vi "main 0.9.2.vi"() -> ()   [LabVIEW 2017]
uses:
  coherent/CH_LM/CH_LM Communication Mode.ctl
  ISEGNHQxxu/iseg NHQ VISA Control.ctl
  <vilib>/Analysis/1siggen.llb/Ramp Pattern by Samples.vi
  <vilib>/Utility/file.llb/Read From Spreadsheet File (DBL).vi
  <vilib>/Instr/_visa.llb/VISA Configure Serial Port (Instr).vi
  Keysight B2980 Series/Public/Data/Read Measurement (Single Point).vi
  Keysight B2980 Series/Public/Configure/Measurement/Configure Current Measurement (Aperture).vi
  <vilib>/Utility/file.llb/Write To Spreadsheet File (DBL).vi
  <vilib>/Utility/file.llb/Write To Spreadsheet File (string).vi
  <vilib>/Platform/browser.llb/Open URL in Default Browser (path).vi
  <vilib>/Analysis/NI_AALBase.lvlib
  coherent/CH_LM.lvlib
  Newport ESP301/Newport ESP301.lvlib
  Keysight B2980 Series/Keysight B2980 Series.lvlib
panel:
  in  "zero":bool
  in  "clear":bool
  in  "Enable Input (F: Disable)":bool
  in  "Enable Output (F: Disable)":bool
  in  "Output Level (0 V)":dbl
  in  "Source Range (20 V)":dbl=20.0
  in  "Aperture Type (1: Medium)":i32(ring)=1 items=["Short", "Medium", "Long"]
  in  "Aperture Integration Time (0.002 s)":dbl=0.002
  in  "Current Range (2E-6 A)":dbl=2e-06
  in  "Auto Current Range (T: Enable)":bool=TRUE
  in  "Auto Current Aperture (T: Enable)":bool=TRUE
  in  "open base path":bool
  in  "Path":path=path "Y:/Ediff/data/2017/01/170106"
  in  "stop":bool
  out "Slide":dbl(slide)=0.99 scale=0.0..1.0
  in  "Tab Control":T1(tab)
  in  "offset":dbl
  out "keysight_graph":cluster{dbl, "mean":dbl}(graph)
  out "esp_pos_fs":dbl caption="[fs]" format="%.6g"
  in  "snap":bool
  in  "dark":bool
  in  "savebin":bool
  in  "savepng":bool
  in  "count?":bool
  in  "dark?":bool=TRUE
  in  "threshold":i32=110
  in  "t_exp":dbl=0.1 caption="exp time [s]"
  in  "dark_load":bool
  in  "frames":i32=100
  in  "avg[t] acc[f]":bool=TRUE
  out "Actual Voltage":dbl[unit]=-0.6 format="%.2f"
  in  "volt_set":bool
  in  "Nominal Voltage":sgl=50.0 max=4000 format="%.2f"
  out "laser power":sgl=6.5658232e-06 format="%^.3e"
  out "Waveform Chart":dbl(graph)=159723533.31
  out "noise-o-meter":dbl=nan format="%.1g"
  in  "array size":i32
  out "[mm]":dbl format="%.6g"
  in  "esp_rel+":bool
  in  "esp_rel-":bool
  in  "esp_abs_go":bool
  in  "esp_rel_delta":dbl=0.1 caption="delta [mm]" min=0.0
  in  "esp_abs_time":dbl caption="[fs]"
  in  "esp_set_t0":bool
  out "t0 @":dbl format="%.6g"
  in  "esp_abs_dest":dbl caption="[mm]"
  in  "Value in":dbl=4.0 caption="binning"
  in  "stats":dbl
  out "x*y":dbl
  in  "x":sgl
  out "Measurement":dbl format="%^#_6g"
  out "e / pulse":dbl
  in  "array size 2":i32
  out "mean":dbl format="%^.2e"
  out "std":dbl format="%^.2e"
  in  "delayscan_go":bool
  in  "waypoints":string[][](table)=[["-100000", "5000"], ["50000", ""], ["", ""]]
  in  "delayscan_header":string="DelayScan01" caption="header"
  in  "iterations":i32
  out "XY Graph":cluster{"Array":dbl[], dbl[]}(graph)
  in  "delayscan_stop":bool
  out "XY Graph 2":cluster{"X":dbl[], "Best Gaussian Fit":dbl[]}[](graph)
  in  "meas_start_power2":bool
  out "meas_voltage":i32=1
  in  "header":string="PowerVoltScan1"
  in  "meas_start_power":bool
  out "meas_power":sgl=6.5658234e-09 format="%.3f"
  in  "powerscan_n":i32
  out "prog":i32
  in  "pause":bool
  in  "Axis":string(combo)
  out "center":dbl
  in  "range+-[nm]":dbl
  in  "n":i32
  in  "rand[t] seq [f]":bool
  in  "zscan?":bool
  out "Slide 2":dbl(slide)=0.999 scale=0.0..1.0
  in  "meas_stop_volt":bool
  in  "meas_start_volt":bool
  in  "head":string="PowerVoltScan1"
  in  "volt_start":dbl format="%0.2f"
  in  "volt_end":dbl=1.0 format="%0.2f"
  in  "volt_samples":i32=128
  in  "move2com":bool
  in  "window2":dbl=10000.0 caption="+/- window" format="%#_6e"
  in  "steps2":u32=21 caption="steps"
  out "XY":dbl[][](graph)
  in  "meas_start_XY":bool
  in  "Axis2":string(combo)="4D Z"
  in  "Axis1":string(combo)="4D Z"
  in  "window1":dbl=10000.0 caption="+/- window" format="%#_6e"
  in  "steps1":u32=21 caption="steps"
  in  "meas_stop_XY":bool
  in  "showcom":bool
  in  "VISA ISEG":refnum<visa-resource-name>="COM6"
  in  "Channel (A)":enum16{"A", "B"}(ring)=enum."B"
  in  "IP address":string="172.24.192.135"
  out "error out":errorcluster
  out "coherent":errorcluster={"status"=TRUE, "code"=-1307, "source"="CH_LM.lvlib:CH_LM FGV Meter Info.vi<ERR>\nMeter index not found.\n\n\n<b>Complete call chain:</b>\r\n     CH_LM.lvlib:CH_LM FGV Meter Info.vi\r\n     CH_LM.lvlib:CH_LM Close.vi\r\n     main 0.9.vi"}
  in  "volt_timeout":u32=6000
  in  "volt_threshold":sgl=2.0 max=4000 format="%.2f"
  in  "esp_axis":i32=2 caption="ESP Axis" min=1 max=3
  in  "esp_visa":refnum<visa-resource-name>="COM1" caption="ESP VISA"
  out "esp301":errorcluster={"status"=TRUE, "code"=-1073807346, "source"="VISA Open in Newport ESP301.lvlib:Initialize.vi->main 0.9.vi"}
  out "response":string
  in  "arduino COM":refnum<visa-resource-name>="COM13"
  in  "arduino_steps":i32
  in  "arduino_go":bool
  out "keysight 2":errorcluster={"status"=TRUE, "code"=-1073807346, "source"="VISA Open in Newport ESP301.lvlib:Initialize.vi->main 0.9.vi"}
  in  "keysight":refnum<visa-resource-name>="USB0::0x0957::0x9418::MY54320162::INSTR"
  in  "Channel (1: Channel 1)":i32(ring)=1 items=["Channel 1"=1, "Channel 2"=2]
  out "captured":dbl[][](graph)
  out "live":dbl[][](graph)
  in  "close":bool
  # "%"
  # "camera"
  # "voltage supply"
  # "delay stage"
  # "absolute"
  # "power meter"
  # "Axis2"
  # "Axis1"
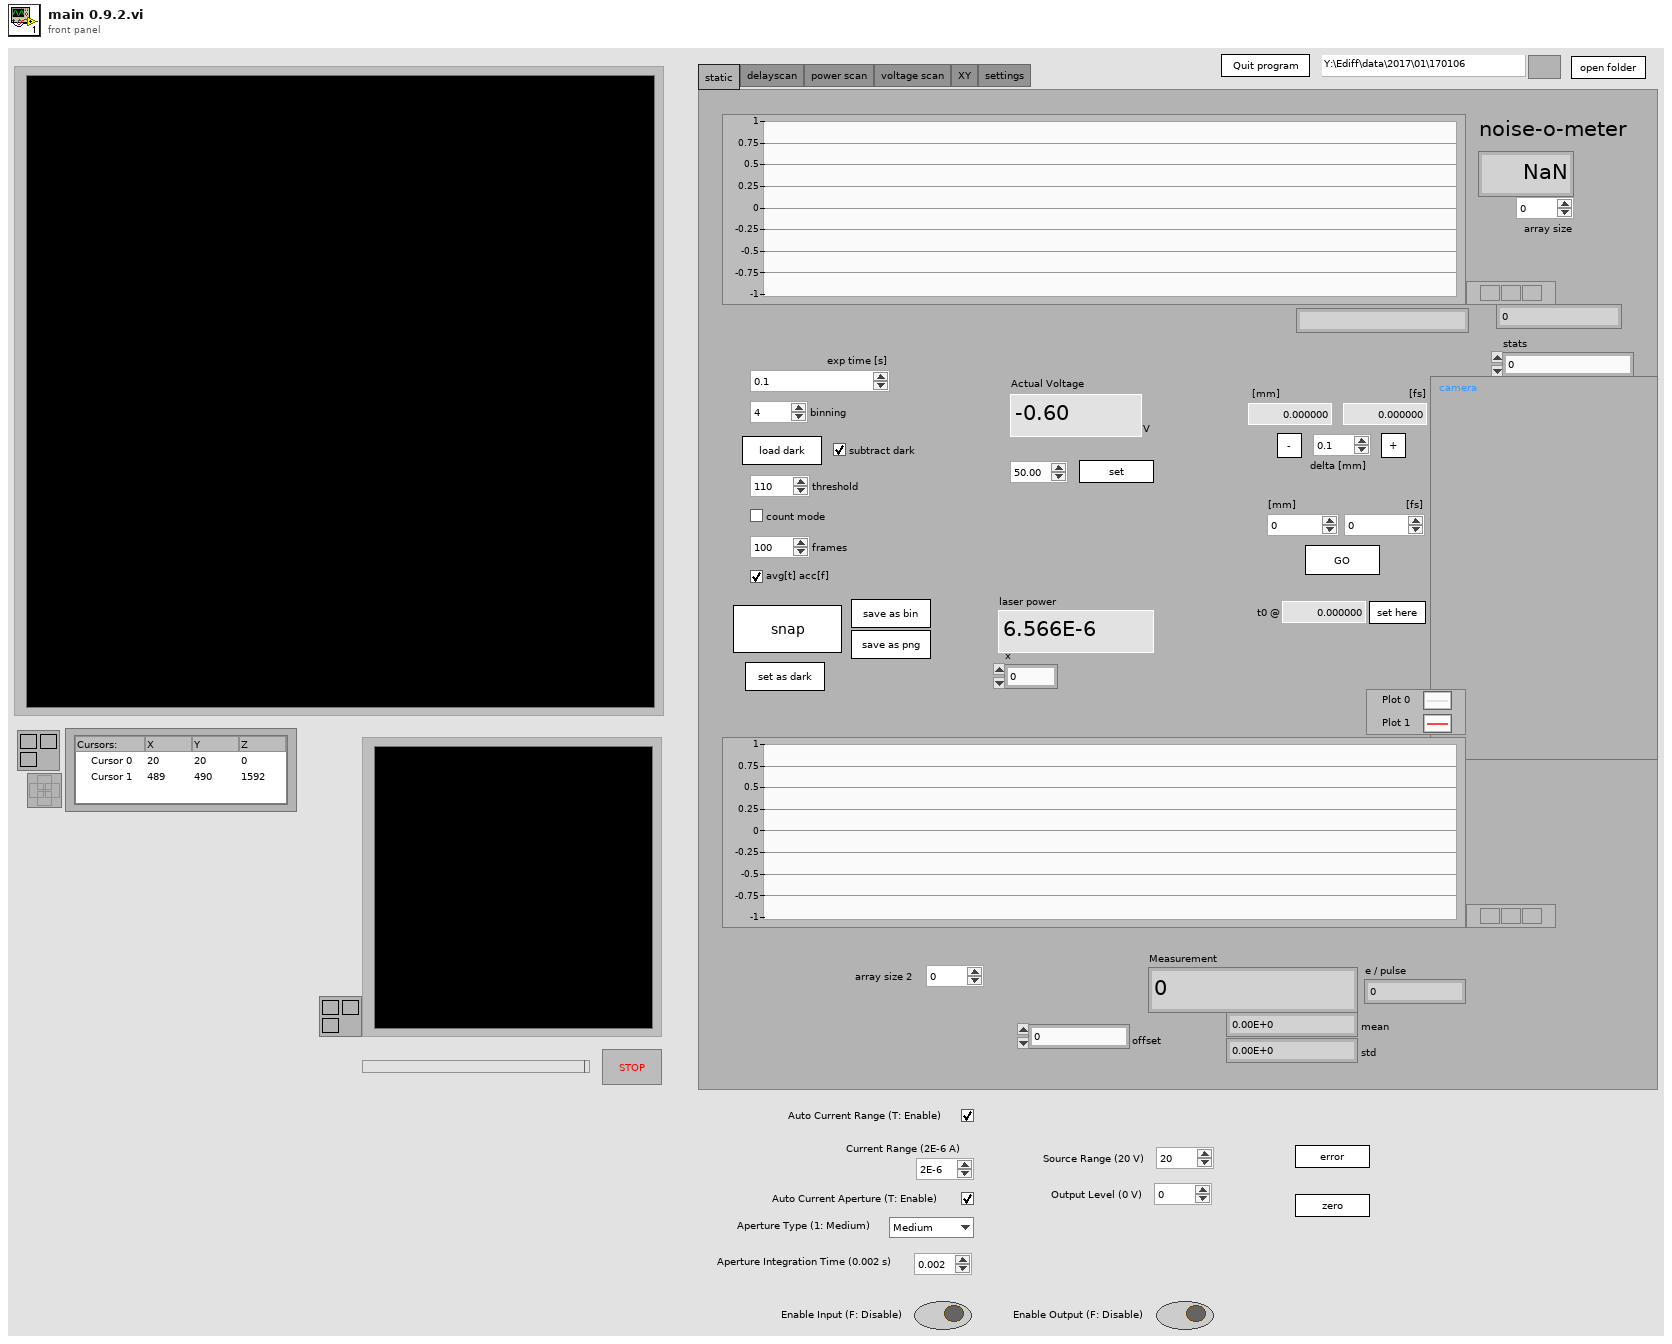
[diagram p1: front panel]
types:
  T1 = enum32{"static", "delayscan", "power scan", "voltage scan", "XY", "settings"}
  T2 = typedef "CH_LM.lvlib/CH_LM Communication Mode.ctl" = enum16{"None", "USB", "GPIB", "RS232"}
  T3 = typedef "Image Type" = u32
  T4 = typedef "IMAQ Image.ctl" = refnum<image>
  T5 = cluster{"height":u32, "width":u32, "datatype":u32}
  T6 = typedef "iseg NHQ VISA Control.ctl" = cluster{"VISA Resource Name":refnum<visa-resource-name>, "FP Notation":bool, "Maximum Voltage":u32, "Maximum Current":u32}
  T7 = typedef "CH_LM.lvlib/CH_LM Streaming Data.ctl" = cluster{"Value":sgl, "Quad Distance":cluster{"X":sgl, "Y":sgl}, "Display Data":cluster{"Format ID":u8, "Scale ID":u8}, "Unit ID":u8, "Flags":u32, "Pulse Period":u32, "Sequence ID":u32, "Unit String":string}
  T8 = cluster{"Axis1 moving":bool, "Axis2 moving":bool, "Axis3 moving":bool, "Axis4 moving":bool, "Motor Power of at least one axis":bool, "Reserved":bool, "Reserved":bool, "Reserved":bool, "Axis5 moving 2":bool, "Axis6 moving 2":bool, "Reserved":bool, "Reserved":bool, "Motor Power of at least one axis":bool, "Reserved":bool, "Reserved":bool, "Reserved":bool}
  T9 = typedef "LVCursorListTypeDef.ctl" = cluster{"Name":string, "Color":u32, "Style":u8, "Point Style":u8, "Name Visible":bool, "Allow Drag":bool, "Cursor Mode":u32, "Plot":i32, "Index":i32, "Position":cluster{"X":dbl, "Y":dbl}, "X Scale":u32, "Y Scale":u32, "Watch Plots":i32[], "Watch All Plots":bool, "Plot Area":i32, "Label Offset":cluster{"X":dbl, "Y":dbl}}[]
  T10 = cluster{"Name":string, "Color":u32, "Style":u8, "Point Style":u8, "Name Visible":bool, "Allow Drag":bool, "Cursor Mode":u32, "Plot":i32, "Index":i32, "Position":cluster{"X":dbl, "Y":dbl}, "X Scale":u32, "Y Scale":u32, "Watch Plots":i32[], "Watch All Plots":bool, "Plot Area":i32, "Label Offset":cluster{"X":dbl, "Y":dbl}}
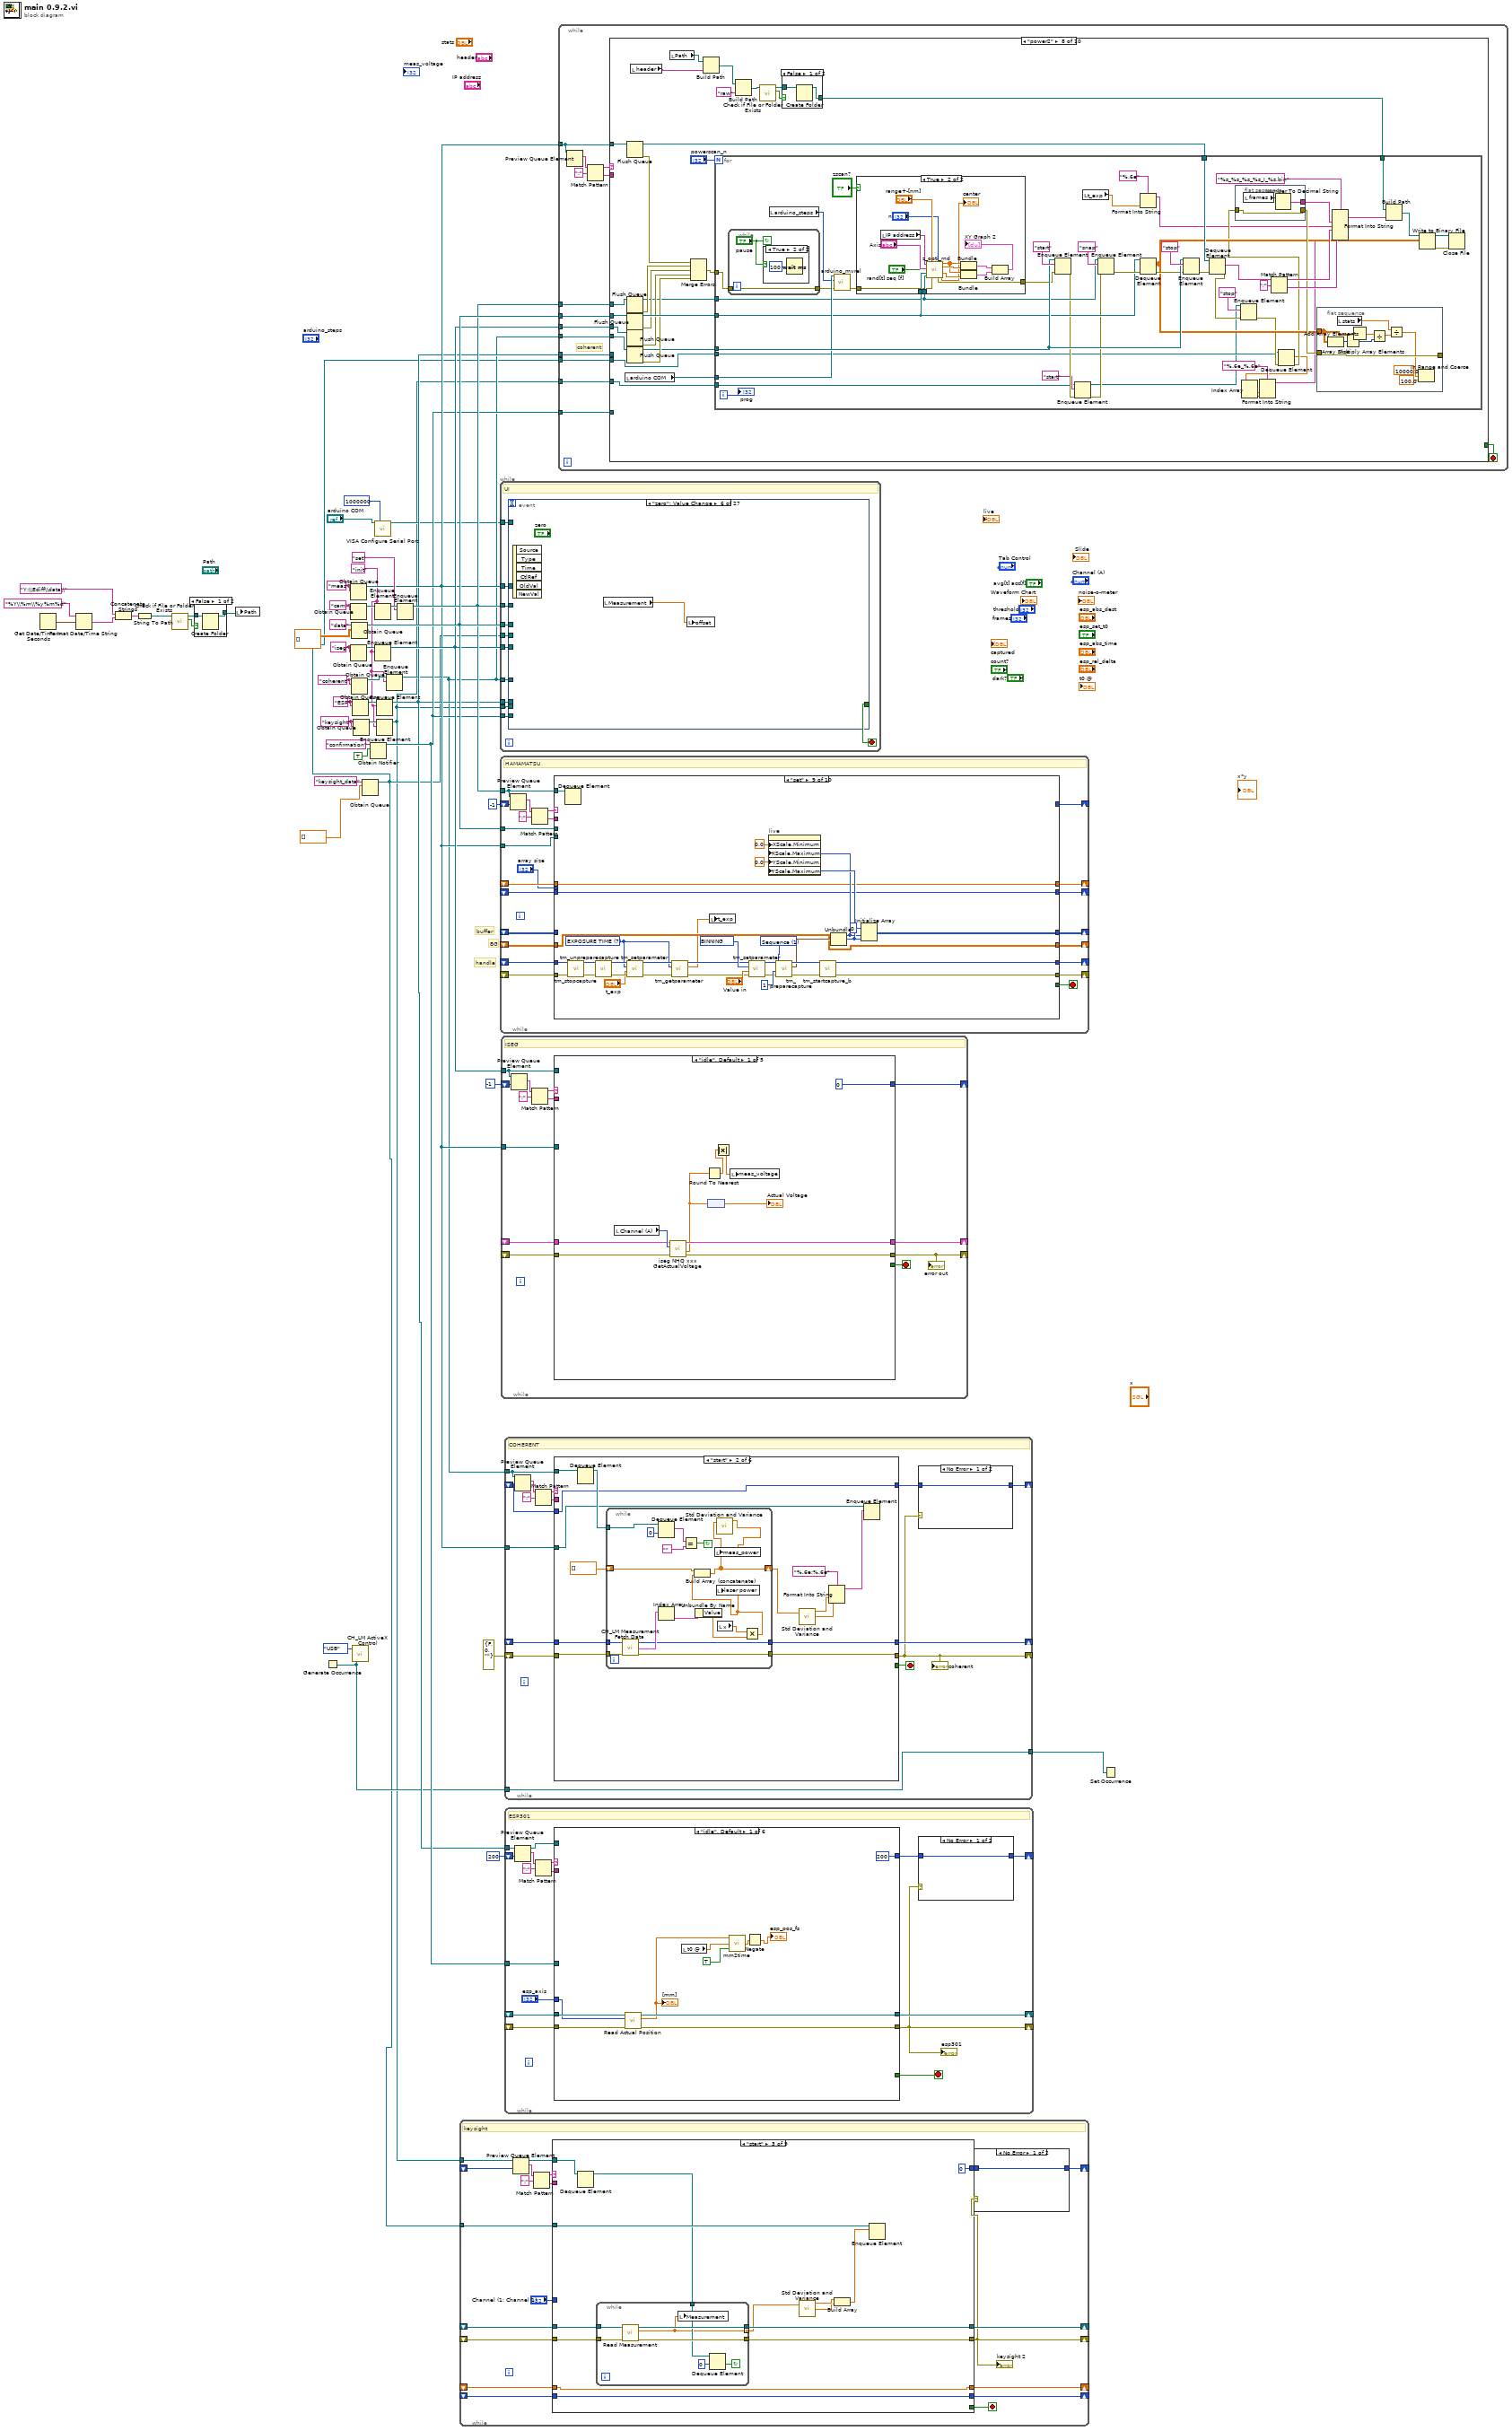
[diagram p0: block diagram]
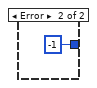
[diagram p2: hidden frame]
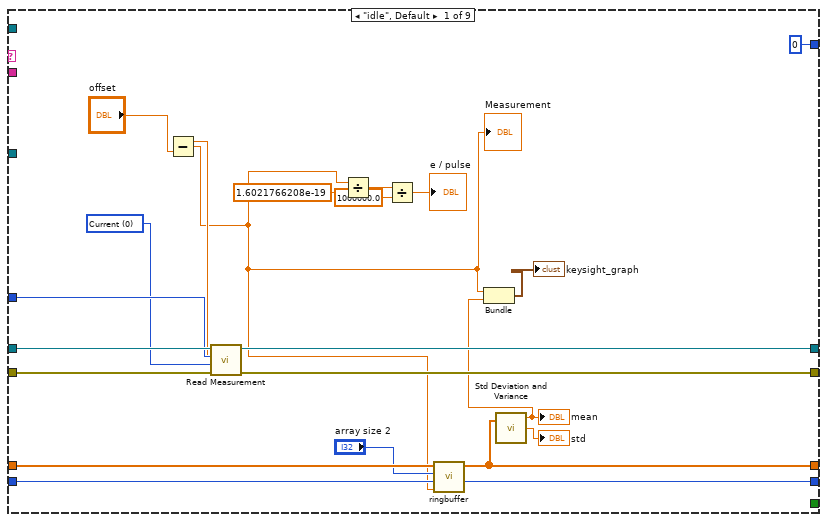
[diagram p3: hidden frame]
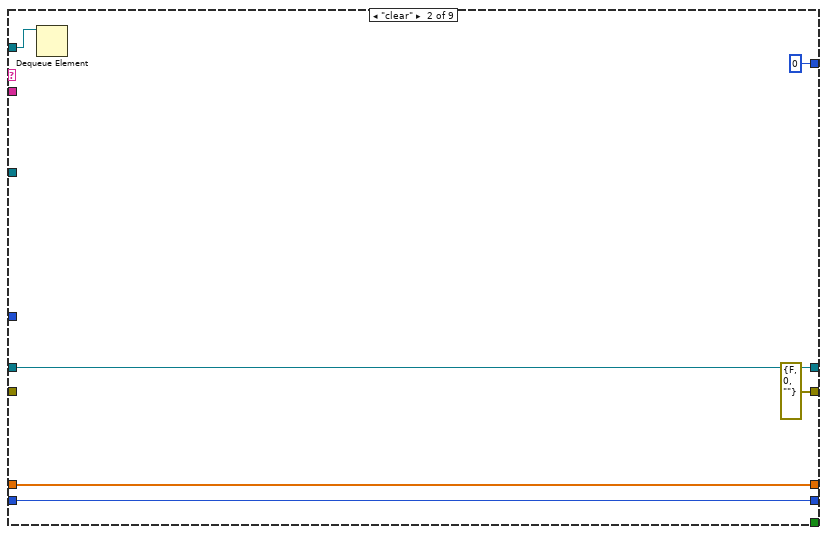
[diagram p4: hidden frame]
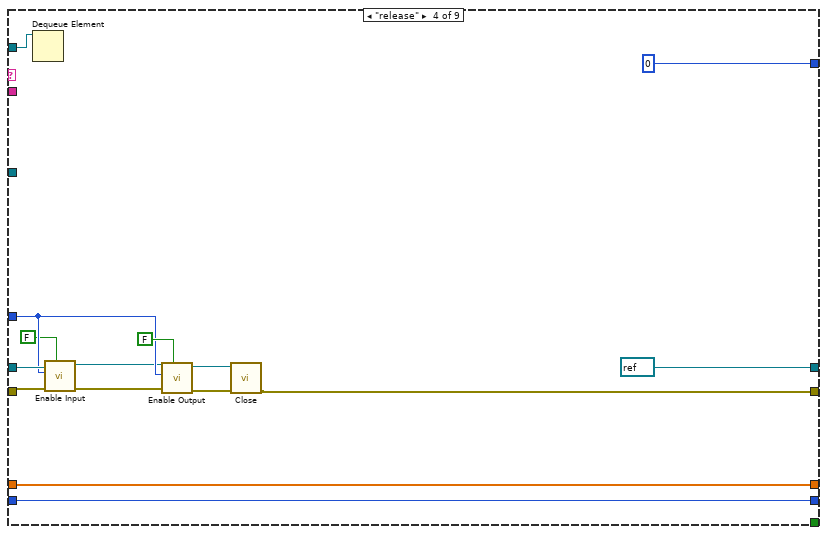
[diagram p5: hidden frame]
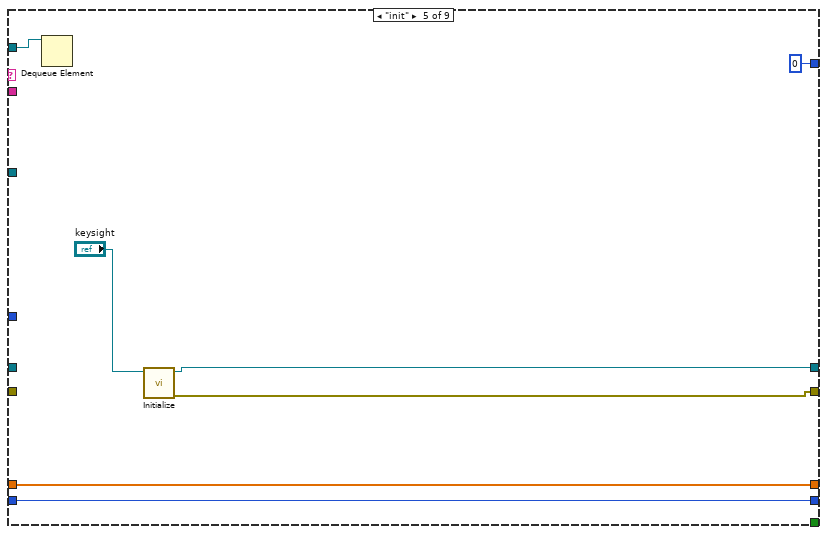
[diagram p6: hidden frame]
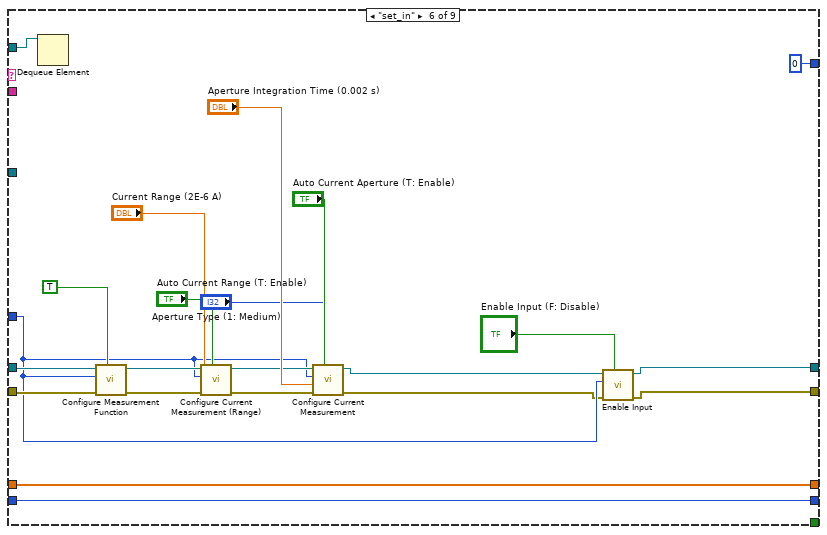
[diagram p7: hidden frame]
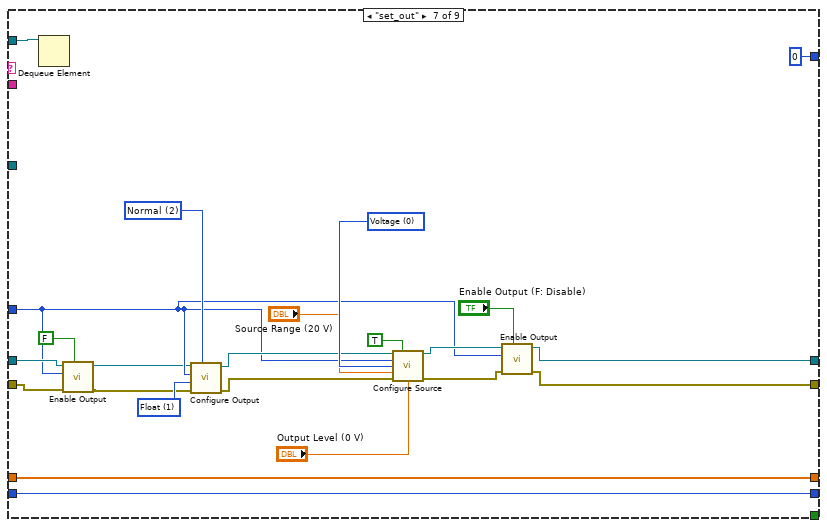
[diagram p8: hidden frame]
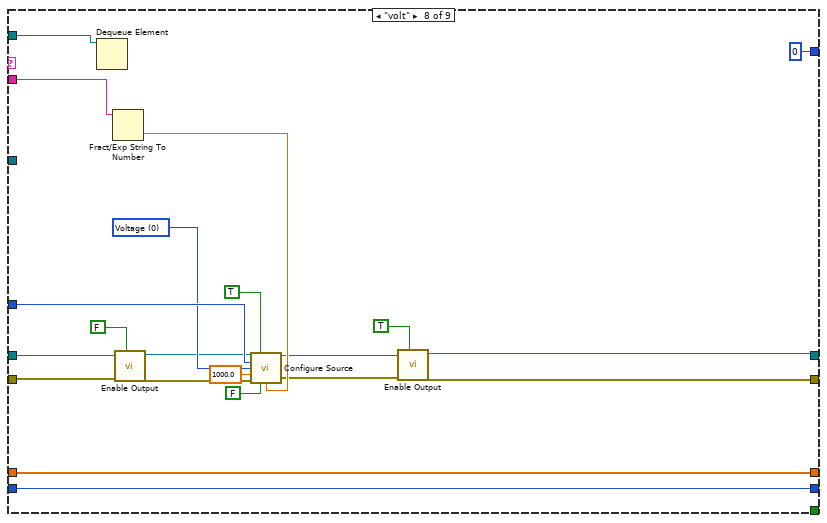
[diagram p9: hidden frame]
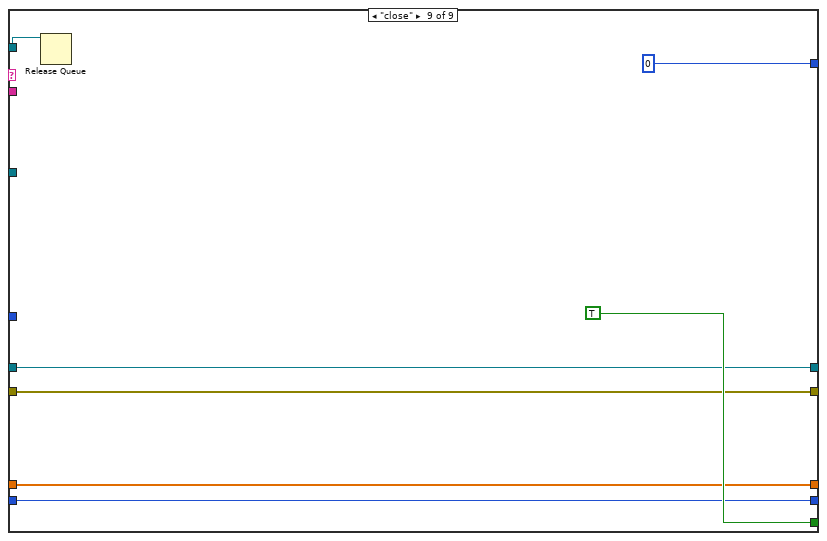
[diagram p10: hidden frame]
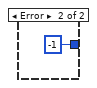
[diagram p12: hidden frame]
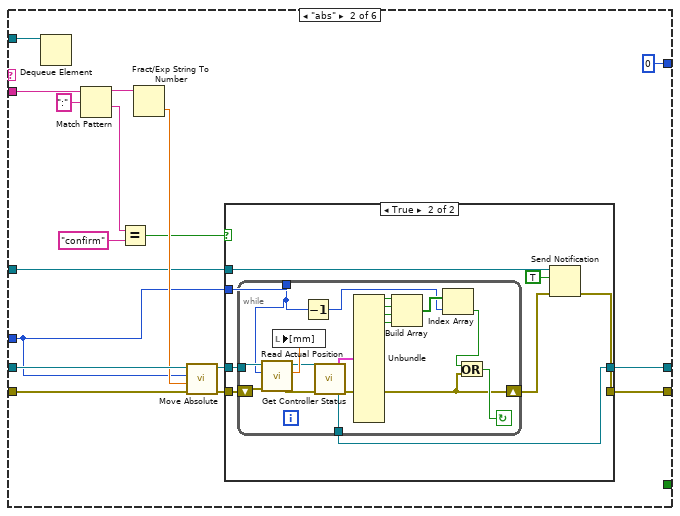
[diagram p13: hidden frame]
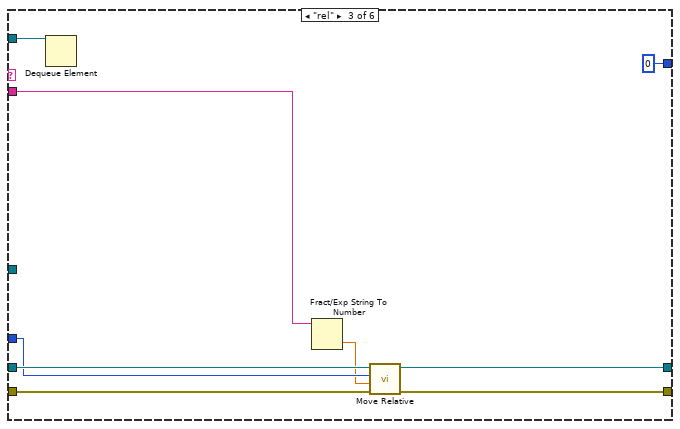
[diagram p15: hidden frame]
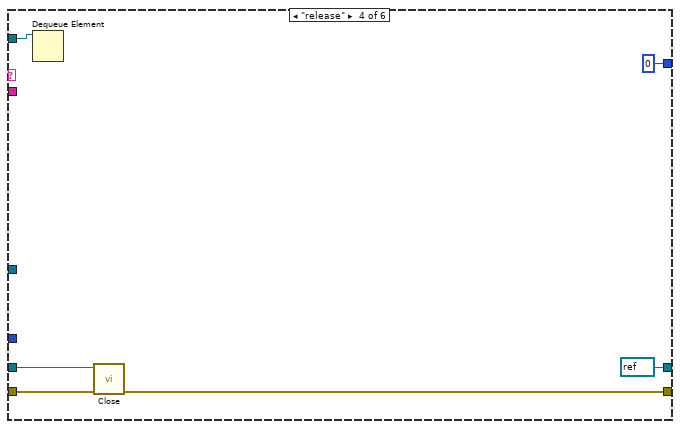
[diagram p16: hidden frame]
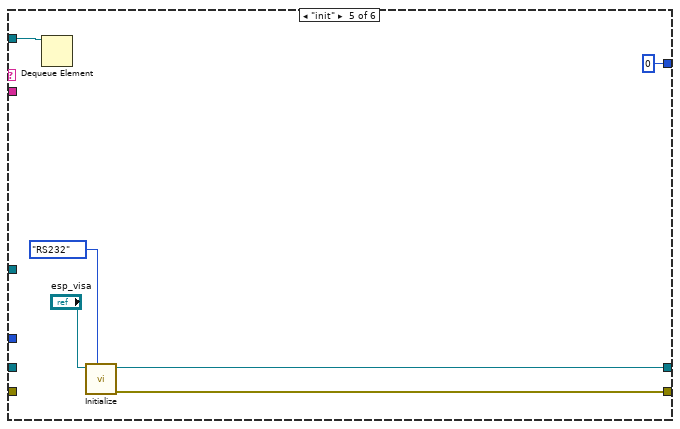
[diagram p17: hidden frame]
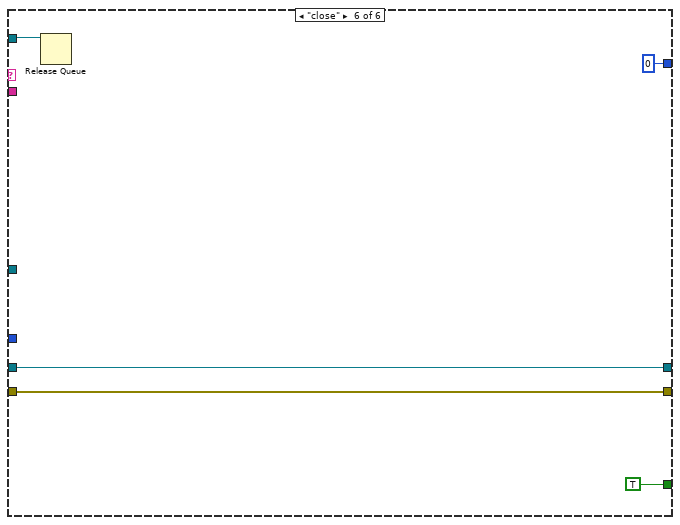
[diagram p18: hidden frame]
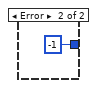
[diagram p19: hidden frame]
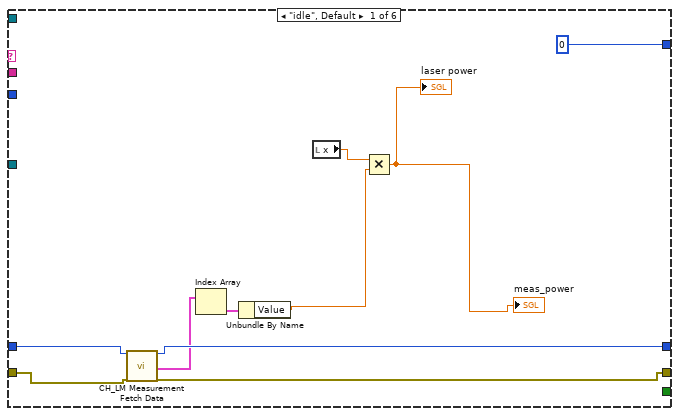
[diagram p20: hidden frame]
diagram:
  w6 = "keysight" ("name (unnamed)")
  w28 = "ESP" ("name (unnamed)")
  w34 = "coherent" ("name (unnamed)")
  w38 = "iseg" ("name (unnamed)")
  w5 = "init" ("element")
  w45 = "meas" ("name (unnamed)")
  w46 = "cam" ("name (unnamed)")
  # "BG"
  # "handle"
  # "buffer"
  n1 = Get Date/Time In Seconds() -> (seconds since 1Jan1904=w25:timestamp)
  n2 = Format Date/Time String(time format string (%c)="%Y\\%m\\%y%m%d", seconds (now)=w25) -> (date/time string=w23:string)  [unwired: 1 in]
  n3 = Concatenate Strings("Y:\\Ediff\\data\\" ("string"), w23) -> (w21:string)
  n4 = String To Path(string=w21) -> (path=w18:path)
  n5 = call <vilib>:"Check if File or Folder Exists.vi"("path"=w18) -> ("file or folder exists?"=w20:bool, "dup path"=w19:path)  [unwired: 8 in, 1 out]
  n6 = case shown="False" w20 {
    tunnel: [w50 w51] -> w17
    tunnel: w19 -> [w49 w51]
    frame False {
      n7 = Create Folder(path (use dialog)=w49) -> (created path=w50:path)  [unwired: 2 in, 2 out]
    }
    frame True {
    }
  }
  n8 = local write "Path"(w17) -> ()
  n9 = Generate Occurrence() -> (w13:refnum<k4>)
  n10 = Obtain Queue(name (unnamed)=w45, element data type=w45) -> (queue out=w32:refnum<queue>)  [unwired: 3 in, 2 out]
  n11 = Obtain Queue(name (unnamed)=w46, element data type=w46) -> (queue out=w48:refnum<queue>)  [unwired: 3 in, 2 out]
  n12 = Obtain Queue(name (unnamed)=w38, element data type=w38) -> (queue out=w37:refnum<queue>)  [unwired: 3 in, 2 out]
  n13 = Obtain Queue(name (unnamed)="data", element data type=dbl[][] []) -> (queue out=w41:refnum<queue>)  [unwired: 3 in, 2 out]
  n14 = Obtain Queue(name (unnamed)=w34, element data type=w34) -> (queue out=w16:refnum<queue>)  [unwired: 3 in, 2 out]
  n15 = Obtain Queue(name (unnamed)=w28, element data type=w28) -> (queue out=w27:refnum<queue>)  [unwired: 3 in, 2 out]
  n16 = call "CH_LM ActiveX Control.vi"("Communication Mode"=CH_LM_Communication_Mode."USB", "MonitorStop Occurrence"=w13) -> ()  [unwired: 3 in, 1 out]
  n17 = Obtain Queue(name (unnamed)=w6, element data type=w6) -> (queue out=w7:refnum<queue>)  [unwired: 3 in, 2 out]
  n18 = Obtain Queue(name (unnamed)="keysight_data", element data type=dbl[] []) -> (queue out=w3:refnum<queue>)  [unwired: 3 in, 2 out]
  n19 = Obtain Notifier(name (unnamed)="confirmation", notification data type=TRUE) -> (notifier out=w29:refnum<notifier>)  [unwired: 2 in, 2 out]
  n20 = call-poly "VISA Configure Serial Port"("VISA resource name"="arduino COM", "timeout (10sec)"=u32 1000000) -> ("VISA resource name out"=w10:refnum<visa-resource-name>)  [unwired: 12 in, 1 out]
  n21 = Enqueue Element(queue=w48, element=w5) -> (queue out=w44:refnum<queue>)  [unwired: 2 in, 2 out]
  n22 = Enqueue Element(queue=w37, element=w5) -> (queue out=w35:refnum<queue>)  [unwired: 2 in, 2 out]
  n23 = Enqueue Element(queue=w27, element=w5) -> (queue out=w26:refnum<queue>)  [unwired: 2 in, 2 out]
  n24 = Enqueue Element(queue=w7, element=w5) -> (queue out=w2:refnum<queue>)  [unwired: 2 in, 2 out]
  n25 = Enqueue Element(queue=w16, element=w5) -> (queue out=w15:refnum<queue>)  [unwired: 2 in, 2 out]
  n26 = Enqueue Element(queue=w44, element="set") -> (queue out=w40:refnum<queue>)  [unwired: 2 in, 2 out]
  n27 = while {
    shift-right: [w60] -> _
    shift-left: _ -> [w66]
    shift-right: [w64] -> _
    shift-left: _ -> [w65]
    shift-right: [w62] -> _
    shift-left: _ -> [w61]
    tunnel: w2 -> [w58]
    tunnel: w3 -> [w56]
    shift-right: [w55] -> _
    shift-left: _ -> [w54]
    shift-right: [w52] -> _
    shift-left: _ -> [w53]
    stop <- w67 stop-if-true
    # "keysight"
    n28 = Preview Queue Element(queue=w58, timeout in ms (-1)=w65) -> (queue out=w63:refnum<queue>, element=w71:string)  [unwired: 1 in, 2 out]
    n29 = Match Pattern(string=w71, regular expression=":") -> (before substring=w69:string, after substring=w68:string)  [unwired: 1 in, 2 out]
    n30 = case shown="\"start\"" w69 {
      tunnel: w68 -> [_ _ _ _ _ _ _ w208 _]
      tunnel: [_ _ _ _ _ _ _ _ TRUE] -> w67
      tunnel: [w91 errorcluster {"status"=FALSE, "code"=0, "source"=""} ("error out") w112 w135 w141 w161 w178 w196 w217] -> w60
      tunnel: w66 -> [w94 _ w114 w130 _ w163 w175 w201 w217]
      tunnel: w63 -> [_ w98 w109 w138 w145 w148 w176 w205 w215]
      tunnel: [w92 w100 w113 refnum<visa-resource-name> refnum ("VISA resource name out") w142 w162 w179 w197 w216] -> w62
      tunnel: w61 -> [w95 w100 w115 w131 _ w164 w174 w204 w216]
      tunnel: [0 0 0 0 0 0 0 0 0] -> w59
      tunnel: "Channel (1: Channel 1)" -> [w93 _ _ w128 _ w153 w173 w211 _]
      tunnel: w56 -> [_ _ w110 _ _ _ _ _ _]
      tunnel: w54 -> [w82 w97 w107 w125 w140 w147 w169 w192 w213]
      tunnel: [w78 w97 w107 w125 w140 w147 w169 w192 w213] -> w55
      tunnel: w53 -> [w81 w96 w106 w124 w139 w146 w168 w191 w212]
      tunnel: [w79 w96 w106 w124 w139 w146 w168 w191 w212] -> w52
      frame "idle", Default {
        w89 = 0 items=["Current", "Status", "Time", "Charge", "Humidity", "Resistance", "Source", "Temperature", "Voltage"] ("Data Type (0: Current)")
        n31 = call-poly "Read Measurement.vi"("error in (no error)"=w94, "Data Type (0: Current)"=w89, "Channel (1: Channel 1)"=w93, "VISA resource name"=w95) -> ("error out"=w91:errorcluster, "Measurement"=w84:dbl, "VISA resource name out"=w92:refnum<visa-resource-name>)  [unwired: 1 in, 4 out]
        n32 = Subtract(x=w84, y="offset") -> (x-y=w75:dbl)
        "Measurement" <- w75
        n33 = Divide(x=w75, y=1.6021766208e-19) -> (x/y=w87:dbl)
        n34 = Divide(x=w87, y=1000000.0) -> (x/y=→"e / pulse":dbl)
        n35 = call "ringbuffer.vi"("new val"=w75, "index in"=w81, "array size"="array size 2", "array in"=w82) -> ("index out"=w79:i32, "array out"=w78:dbl[])  [unwired: 6 in]
        n36 = call <vilib>:"Std Deviation and Variance.vi"("X"=w78) -> ("mean"=w76:dbl, "standard deviation"=→"std":dbl)  [unwired: 1 in, 1 out]
        "mean" <- w76
        n37 = Bundle(w75, "mean"=w76) -> (→"keysight_graph":cluster{dbl, "mean":dbl})  [unwired: 1 in]
      }
      frame "clear" {
        n38 = Dequeue Element(queue=w98) -> ()  [unwired: 2 in, 4 out]
      }
      frame "start" {
        n39 = Dequeue Element(queue=w109) -> (queue out=w108:refnum<queue>)  [unwired: 2 in, 3 out]
        n40 = while {
          tunnel: w115 -> [w123]
          tunnel: w114 -> [w122]
          tunnel: [w121] -> w113
          tunnel: [w120] -> w112
          tunnel: w108 -> [w117]
          tunnel: [w116] -> w105 mode=indexing
          stop <- w118 continue-if-true
          n41 = call-poly "Read Measurement.vi"("error in (no error)"=w122, "VISA resource name"=w123) -> ("error out"=w120:errorcluster, "Measurement"=w116:dbl, "VISA resource name out"=w121:refnum<visa-resource-name>)  [unwired: 3 in, 4 out]
          n42 = local write "Measurement"(w116) -> ()
          n43 = Dequeue Element(queue=w117, timeout in ms (-1)=0) -> (timed out?=w118:bool)  [unwired: 1 in, 3 out]
        }
        n44 = call <vilib>:"Std Deviation and Variance.vi"("X"=w105) -> ("mean"=w104:dbl, "standard deviation"=w103:dbl)  [unwired: 1 in, 1 out]
        n45 = Build Array(w104, w103) -> (w102:dbl[])
        n46 = Enqueue Element(queue=w110, element=w102) -> ()  [unwired: 2 in, 3 out]
      }
      frame "release" {
        n47 = Dequeue Element(queue=w138) -> ()  [unwired: 2 in, 4 out]
        n48 = call "Enable Input.vi"("Enable Input (F: Disable)"=FALSE, "error in (no error)"=w130, "Channel (1: Channel 1)"=w128, "VISA resource name"=w131) -> ("error out"=w129:errorcluster, "VISA resource name out"=w126:refnum<visa-resource-name>)  [unwired: 5 in, 1 out]
        n49 = call "Enable Output.vi"("Enable Output (F: Disable)"=FALSE, "error in (no error)"=w129, "Channel (1: Channel 1)"=w128, "VISA resource name"=w126) -> ("error out"=w133:errorcluster, "VISA resource name out"=w134:refnum<visa-resource-name>)  [unwired: 5 in, 1 out]
        n50 = call "Close.vi"("error in (no error)"=w133, "VISA resource name"=w134) -> ("error out"=w135:errorcluster)  [unwired: 9 out]
      }
      frame "init" {
        n51 = Dequeue Element(queue=w145) -> ()  [unwired: 2 in, 4 out]
        n52 = call "Initialize.vi"("VISA resource name"="keysight") -> ("error out"=w141:errorcluster, "VISA resource name out"=w142:refnum<visa-resource-name>)  [unwired: 4 in, 5 out]
      }
      frame "set_in" {
        n53 = Dequeue Element(queue=w148) -> ()  [unwired: 2 in, 4 out]
        n54 = call "Configure Measurement Function.vi"("Enable Current Measurement (T: Enable)"=TRUE, "error in (no error)"=w163, "Channel (1: Channel 1)"=w153, "VISA resource name"=w164) -> ("error out"=w165:errorcluster, "VISA resource name out"=w166:refnum<visa-resource-name>)  [unwired: 3 in, 3 out]
        n55 = call "Configure Current Measurement (Range).vi"("Auto Current Range (T: Enable)"="Auto Current Range (T: Enable)", "error in (no error)"=w165, "Current Range (2E-6 A)"="Current Range (2E-6 A)", "Channel (1: Channel 1)"=w153, "VISA resource name"=w166) -> ("error out"=w154:errorcluster, "VISA resource name out"=w155:refnum<visa-resource-name>)  [unwired: 2 in, 3 out]
        n56 = call-poly "Configure Current Measurement.vi"("Aperture Type (1: Medium)"="Aperture Type (1: Medium)", "Auto Current Aperture (T: Enable)"="Auto Current Aperture (T: Enable)", "error in (no error)"=w154, "Aperture Integration Time (0.002 s)"="Aperture Integration Time (0.002 s)", "Channel (1: Channel 1)"=w153, "VISA resource name"=w155) -> ("error out"=w151:errorcluster, "VISA resource name out"=w152:refnum<visa-resource-name>)  [unwired: 4 in]
        n57 = call "Enable Input.vi"("Enable Input (F: Disable)"="Enable Input (F: Disable)", "error in (no error)"=w151, "Channel (1: Channel 1)"=w153, "VISA resource name"=w152) -> ("error out"=w161:errorcluster, "VISA resource name out"=w162:refnum<visa-resource-name>)  [unwired: 5 in, 1 out]
      }
      frame "set_out" {
        w190 = 0 items=["Voltage"] ("Source Type (0: Voltage)")
        w188 = 2 items=["Zero", "HIZ", "Normal"] ("Source Condition (2: Normal)")
        w189 = 1 items=["Common", "Float"] ("Low Terminal State (1: Float)")
        n58 = Dequeue Element(queue=w176) -> ()  [unwired: 2 in, 4 out]
        n59 = call "Enable Output.vi"("Enable Output (F: Disable)"=FALSE, "error in (no error)"=w175, "Channel (1: Channel 1)"=w173, "VISA resource name"=w174) -> ("error out"=w170:errorcluster, "VISA resource name out"=w171:refnum<visa-resource-name>)  [unwired: 5 in, 1 out]
        n60 = call "Configure Output.vi"("Source Condition (2: Normal)"=w188, "error in (no error)"=w170, "Low Terminal State (1: Float)"=w189, "Channel (1: Channel 1)"=w173, "VISA resource name"=w171) -> ("error out"=w186:errorcluster, "VISA resource name out"=w187:refnum<visa-resource-name>)  [unwired: 5 in]
        n61 = call "Configure Source.vi"("VISA resource name"=w187, "Enable Continuous Output (F: Disable)"=TRUE, "Channel (1: Channel 1)"=w173, "Source Type (0: Voltage)"=w190, "Source Range (20 V)"="Source Range (20 V)", "error in (no error)"=w186, "Output Level (0 V)"="Output Level (0 V)") -> ("VISA resource name out"=w182:refnum<visa-resource-name>, "error out"=w181:errorcluster)  [unwired: 7 in]
        n62 = call "Enable Output.vi"("Enable Output (F: Disable)"="Enable Output (F: Disable)", "error in (no error)"=w181, "Channel (1: Channel 1)"=w173, "VISA resource name"=w182) -> ("error out"=w178:errorcluster, "VISA resource name out"=w179:refnum<visa-resource-name>)  [unwired: 5 in, 1 out]
      }
      frame "volt" {
        w210 = 0 items=["Voltage"] ("Source Type (0: Voltage)")
        n63 = Dequeue Element(queue=w205) -> ()  [unwired: 2 in, 4 out]
        n64 = Fract/Exp String To Number(string=w208) -> (number=w207:dbl)  [unwired: 3 in, 1 out]
        n65 = call "Enable Output.vi"("Enable Output (F: Disable)"=FALSE, "error in (no error)"=w201, "VISA resource name"=w204) -> ("error out"=w202:errorcluster, "VISA resource name out"=w203:refnum<visa-resource-name>)  [unwired: 6 in, 1 out]
        n66 = call "Configure Source.vi"("VISA resource name"=w203, "Enable Continuous Output (F: Disable)"=TRUE, "Channel (1: Channel 1)"=w211, "Source Type (0: Voltage)"=w210, "Source Range (20 V)"=1000.0, "error in (no error)"=w202, "Enable Resistive Limit (F: Disable)"=FALSE, "Output Level (0 V)"=w207) -> ("VISA resource name out"=w199:refnum<visa-resource-name>, "error out"=w198:errorcluster)  [unwired: 6 in]
        n67 = call "Enable Output.vi"("Enable Output (F: Disable)"=TRUE, "error in (no error)"=w198, "VISA resource name"=w199) -> ("error out"=w196:errorcluster, "VISA resource name out"=w197:refnum<visa-resource-name>)  [unwired: 6 in, 1 out]
      }
      frame "close" {
        n68 = Release Queue(queue=w215) -> ()  [unwired: 2 in, 3 out]
      }
    }
    "keysight 2" <- w60
    n69 = case shown="No Error" w60 {
      tunnel: [w72 -1] -> w64
      tunnel: w59 -> [w72 _]
      frame No Error {
      }
      frame Error {
      }
    }
  }
  n70 = while {
    tunnel: w40 -> [w229]
    tunnel: w32 -> [w228]
    tunnel: w41 -> [w227]
    tunnel: w35 -> [w225]
    tunnel: w15 -> [w224]
    tunnel: w29 -> [w223]
    tunnel: w26 -> [w222]
    tunnel: w10 -> [w221]
    tunnel: w2 -> [w220]
    tunnel: w3 -> [w219]
    stop <- w226 stop-if-true
    # "UI"
    n71 = event shown="[5] \"zero\": Value Change" {
      selector: _ -> [_ _ _ _ _ _ _ _ _ _ _ _ _ _ _ _ _ _ _ _ _ _ _ _ _ _ _]
      dyn-events: _ -> [_ _ _ _ _ _ _ _ _ _ _ _ _ _ _ _ _ _ _ _ _ _ _ _ _ _ _]
      timeout: _ -> [_ _ _ _ _ _ _ _ _ _ _ _ _ _ _ _ _ _ _ _ _ _ _ _ _ _ _]
      tunnel: w229 -> [_ w245 _ _ _ _ _ _ _ _ _ _ w282 w284 _ _ _ _ _ _ _ _ _ w342 _ _ _]
      tunnel: w228 -> [_ w246 _ _ _ _ _ _ _ _ w275 _ _ _ w285 w288 w289 w292 w293 _ _ _ w336 _ w349 w351 _]
      tunnel: w227 -> [_ _ _ _ _ _ _ _ _ _ _ _ _ _ _ _ _ _ _ _ _ _ _ _ _ _ _]
      tunnel: [_ TRUE _ _ _ _ _ _ _ _ _ _ _ _ _ _ _ _ _ _ _ _ _ _ _ _ _] -> w226
      tunnel: w225 -> [_ w242 _ _ _ _ _ _ _ _ _ _ _ _ _ _ _ _ _ _ _ _ _ _ _ _ w356]
      tunnel: w224 -> [_ w239 _ _ _ _ _ _ _ _ _ _ _ _ _ _ _ _ _ _ _ _ _ _ _ _ _]
      tunnel: w223 -> [_ w236 _ _ _ _ _ _ _ _ _ _ _ _ _ _ _ _ _ _ _ _ _ _ _ _ _]
      tunnel: w222 -> [_ w238 _ _ _ _ w259 w264 _ _ _ _ _ _ _ _ _ _ _ _ _ _ _ _ _ _ _]
      tunnel: w221 -> [_ w235 _ _ _ _ _ _ _ _ _ _ _ _ _ _ _ _ _ w296 _ _ _ _ _ _ _]
      tunnel: w220 -> [_ w230 w248 w249 w251 _ _ _ _ _ _ _ _ _ _ _ _ _ _ _ _ _ _ _ _ _ _]
      tunnel: w219 -> [_ _ _ _ _ _ _ _ _ _ _ _ _ _ _ _ _ _ _ _ _ _ _ _ _ _ _]
      event Timeout {
        n72 = event-data() -> ()  [unwired: 1 in, 1 out]
      }
      event "close": Value Change {
        w233 = "close" ("element")
        w234 = "release" ("element")
        n73 = event-data() -> ()  [unwired: 1 in, 1 out]
        n74 = VISA Close(VISA resource name=w235) -> ()  [unwired: 1 in, 1 out]
        n75 = Enqueue Element(queue=w239, element=w234) -> (queue out=w240:refnum<queue>)  [unwired: 2 in, 2 out]
        n76 = Enqueue Element(queue=w238, element=w234) -> (queue out=w237:refnum<queue>)  [unwired: 2 in, 2 out]
        n77 = Enqueue Element(queue=w242, element=w234) -> (queue out=w241:refnum<queue>)  [unwired: 2 in, 2 out]
        n78 = Enqueue Element(queue=w245, element=w234) -> (queue out=w244:refnum<queue>)  [unwired: 2 in, 2 out]
        n79 = Enqueue Element(queue=w246, element=w233) -> ()  [unwired: 2 in, 3 out]
        n80 = Enqueue Element(queue=w244, element=w233) -> ()  [unwired: 2 in, 3 out]
        n81 = Enqueue Element(queue=w241, element=w233) -> ()  [unwired: 2 in, 3 out]
        n82 = Enqueue Element(queue=w240, element=w233) -> ()  [unwired: 2 in, 3 out]
        n83 = Enqueue Element(queue=w237, element=w233) -> ()  [unwired: 2 in, 3 out]
        n84 = Release Notifier(notifier=w236) -> ()  [unwired: 2 in, 3 out]
        n85 = Flush Queue(queue=w230) -> (queue out=w231:refnum<queue>)  [unwired: 1 in, 2 out]
        n86 = Enqueue Element(queue=w231, element=w234) -> (queue out=w232:refnum<queue>)  [unwired: 2 in, 2 out]
        n87 = Enqueue Element(queue=w232, element=w233) -> ()  [unwired: 2 in, 3 out]
      }
      event "Enable Input (F: Disable)", "Aperture Type (1: Medium)", "Aperture Integration Time (0.002 s)", "Current Range (2E-6 A)", "Auto Current Range (T: Enable)", "Auto Current Aperture (T: Enable)": Value Change {
        n88 = event-data() -> ()  [unwired: 1 in, 6 out]
        n89 = Enqueue Element(queue=w248, element="set_in" ("string")) -> ()  [unwired: 2 in, 3 out]
      }
      event "Enable Output (F: Disable)", "Output Level (0 V)", "Source Range (20 V)": Value Change {
        n90 = event-data() -> ()  [unwired: 1 in, 6 out]
        n91 = Enqueue Element(queue=w249, element="set_out" ("string")) -> ()  [unwired: 2 in, 3 out]
      }
      event "clear": Value Change {
        n92 = event-data() -> ()  [unwired: 1 in, 6 out]
        n93 = Enqueue Element(queue=w251, element="clear" ("string")) -> ()  [unwired: 2 in, 3 out]
      }
      event "zero": Value Change {
        n94 = event-data() -> ()  [unwired: 1 in, 6 out]
        n95 = local read "Measurement"() -> (w253:dbl)
        n96 = local write "offset"(w253) -> ()
      }
      event "esp_abs_go": Value Change {
        n97 = event-data() -> ()  [unwired: 1 in, 1 out]
        n98 = local read "esp_abs_dest"() -> (w255:dbl)
        n99 = Number To Fractional String(number=w255) -> (F-format string=w256:string)  [unwired: 3 in]
        n100 = Concatenate Strings("abs:" ("string"), w256, ":confirm" ("string")) -> (w258:string)
        n101 = Enqueue Element(queue=w259, element=w258) -> ()  [unwired: 2 in, 3 out]
      }
      event "esp_rel+", "esp_rel-": Value Change {
        n102 = event-data() -> ()  [unwired: 1 in, 1 out]
        n103 = local read "esp_rel_delta"() -> (w261:dbl)
        n104 = Negate(x=w261) -> (-x=w262:dbl)
        n105 = Select(t=w262, s="esp_rel-", f=w261) -> (s? t:f=w260:dbl)
        n106 = Number To Fractional String(number=w260) -> (F-format string=w266:string)  [unwired: 3 in]
        n107 = Concatenate Strings("rel:" ("string"), w266) -> (w265:string)
        n108 = Enqueue Element(queue=w264, element=w265) -> ()  [unwired: 2 in, 3 out]
      }
      event "esp_set_t0": Value Change {
        n109 = event-data() -> ()  [unwired: 1 in, 1 out]
        n110 = local read "[mm]"() -> (w268:dbl)
        n111 = local write "t0 @"(w268) -> ()
      }
      event "esp_abs_time": Value Change {
        n112 = event-data() -> ()  [unwired: 1 in, 1 out]
        n113 = local read "esp_abs_time"() -> (w270:dbl)
        n114 = local read "t0 @"() -> (w271:dbl)
        n115 = Negate(x=w270) -> (-x=w269:dbl)
        n116 = call "time2mm.vi"("fs[1]/ps[0]"=TRUE, "Offset (mm)"=w271, "time"=w269) -> ("position (mm)"=w272:dbl)
        n117 = local write "esp_abs_dest"(w272) -> ()
      }
      event "delayscan_go": Value Change {
        n118 = event-data() -> ()  [unwired: 1 in, 1 out]
        n119 = Enqueue Element(queue=w275, element="delay") -> ()  [unwired: 2 in, 3 out]
      }
      event "esp_abs_dest": Value Change {
        n120 = event-data() -> ()  [unwired: 1 in, 1 out]
        n121 = local read "esp_abs_dest"() -> (w280:dbl)
        n122 = local read "t0 @"() -> (w279:dbl)
        n123 = call "mm2time.vi"("fs?"=TRUE, "Offset (mm)"=w279, "distance (mm)"=w280) -> ("time in fs/ps seconds"=w277:dbl)
        n124 = Negate(x=w277) -> (-x=w276:dbl)
        n125 = local write "esp_abs_time"(w276) -> ()
      }
      event "dark": Value Change {
        n126 = event-data() -> ()  [unwired: 1 in, 1 out]
        n127 = Enqueue Element(queue=w282, element="dark") -> ()  [unwired: 2 in, 3 out]
      }
      event "t_exp": Value Change {
        n128 = event-data() -> ()  [unwired: 1 in, 1 out]
        n129 = Enqueue Element(queue=w284, element="set") -> ()  [unwired: 2 in, 3 out]
      }
      event "snap": Value Change {
        n130 = event-data() -> ()  [unwired: 1 in, 1 out]
        n131 = Enqueue Element(queue=w285, element="single") -> ()  [unwired: 2 in, 3 out]
      }
      event "meas_start_volt": Value Change {
        n132 = event-data() -> ()  [unwired: 1 in, 1 out]
        n133 = Enqueue Element(queue=w288, element="volt") -> ()  [unwired: 2 in, 3 out]
      }
      event "meas_stop_volt": Value Change {
        n134 = event-data() -> ()  [unwired: 1 in, 1 out]
        n135 = Enqueue Element(queue=w289, element="stop") -> ()  [unwired: 2 in, 3 out]
      }
      event "meas_start_power": Value Change {
        n136 = event-data() -> ()  [unwired: 1 in, 1 out]
        n137 = Enqueue Element(queue=w292, element="power") -> ()  [unwired: 2 in, 3 out]
      }
      event "meas_start_power2": Value Change {
        n138 = event-data() -> ()  [unwired: 1 in, 1 out]
        n139 = Enqueue Element(queue=w293, element="power2") -> ()  [unwired: 2 in, 3 out]
      }
      event "arduino_go": Value Change {
        n140 = event-data() -> ()  [unwired: 1 in, 1 out]
        n141 = local read "arduino_steps"() -> (w297:i32)
        n142 = call "arduino_mvrel.vi"("steps"=w297, "VISA input"=w296) -> ("response"=→"response":string)  [unwired: 7 in, 2 out]
      }
      event "open base path": Value Change {
        n143 = event-data() -> ()  [unwired: 1 in, 1 out]
        n144 = local read "Path"() -> (w298:path)
        n145 = call-poly <vilib>:"Open URL in Default Browser.vi"("path"=w298) -> ()  [unwired: 5 in, 2 out]
      }
      event "savebin", "savepng": Value Change {
        n146 = event-data() -> ()  [unwired: 1 in, 1 out]
        n147 = Get Date/Time In Seconds() -> (seconds since 1Jan1904=w304:timestamp)
        n148 = local read "Path"() -> (w300:path)
        n149 = Format Date/Time String(time format string (%c)="MCPIMG_%Y%m%d_%H%M%S", seconds (now)=w304) -> (date/time string=w299:string)  [unwired: 1 in]
        n150 = local read "captured"() -> (w301:dbl[][])
        n151 = case shown="False" "savebin" {
          tunnel: w301 -> [w319 w335]
          tunnel: w300 -> [w316 w329]
          tunnel: w299 -> [w314 w330]
          frame False {
            w324 = T3 7 items=["Grayscale (U8)", "Grayscale (I16)", "Grayscale (SGL)", "Complex (CSG)", "RGB (U32)", "HSL (U32)", "RGB (U64)", "Grayscale (U16)"] ("Image Type")
            n152 = for {
              tunnel: w319 -> [w327] mode=indexing
              tunnel: [w326] -> w318 mode=indexing
              n153 = Reverse 1D Array(array=w327) -> (reversed array=w326:dbl[])
            }
            n154 = Concatenate Strings(w314, ".png" ("string")) -> (w315:string)
            n155 = Transpose 2D Array(2D array=w318) -> (transposed array=w307:dbl[][])
            n156 = Array Max & Min(array=w307) -> (min value=w306:dbl)  [unwired: 3 out]
            n157 = Build Path(base path=w316, name or relative path=w315) -> (appended path=w317:path)
            n158 = Subtract(x=w307, y=w306) -> (x-y=w305:dbl[][])
            n159 = call "IMAQ Create"("Image Name"="untitled", "Image Type"=w324) -> ("New Image"=w325:T4)  [unwired: 3 in, 1 out]
            n160 = Array Max & Min(array=w305) -> (max value=w312:dbl)  [unwired: 3 out]
            n161 = Divide(x=w305, y=w312) -> (x/y=w311:dbl[][])
            n162 = Multiply(x=w311, y=255) -> (x*y=w309:dbl[][])
            n163 = To Unsigned Word Integer(number=w309) -> (unsigned 16bit integer=w308:u16[][])
            n164 = call "IMAQ ArrayToImage"("Image Pixels (U16)"=w308, "Image"=w325) -> ("Image Out"=w323:T4)  [unwired: 8 in, 1 out]
            n165 = call-poly "IMAQ Write File 2"("Image Quality"=u32 1000, "File Path"=w317, "Image"=w323) -> ("Image Out (duplicate)"=w321:T4)  [unwired: 7 in, 1 out]
            n166 = call "IMAQ Dispose"("Image"=w321) -> ()  [unwired: 5 in, 1 out]
          }
          frame True {
            n167 = Concatenate Strings(w330, ".bin" ("string")) -> (w332:string)
            n168 = Build Path(base path=w329, name or relative path=w332) -> (appended path=w328:path)
            n169 = Write to Binary File(file (use dialog)=w328, data=w335) -> (refnum out=w334:refnum<file>, error out=w333:errorcluster)  [unwired: 4 in, 1 out]
            n170 = Close File(refnum=w334, error in=w333) -> ()  [unwired: 2 out]
          }
        }
      }
      event "meas_start_XY": Value Change {
        n171 = event-data() -> ()  [unwired: 1 in, 1 out]
        n172 = Enqueue Element(queue=w336, element="XY") -> ()  [unwired: 2 in, 3 out]
      }
      event "dark_load": Value Change {
        n173 = event-data() -> ()  [unwired: 1 in, 1 out]
        n174 = local read "Path"() -> (w341:path)
        n175 = call "File Dialog"("start path"=w341) -> ("selected path"=w339:path, "cancelled"=w338:bool)  [unwired: 11 in, 2 out]
        n176 = case shown="False" w338 {
          tunnel: w342 -> [w347 _]
          tunnel: "dark_load:" ("element") -> [w345 _]
          tunnel: w339 -> [w343 _]
          frame False {
            n177 = Path To String(path=w343) -> (string=w344:string)
            n178 = Concatenate Strings(w345, w344) -> (w346:string)
            n179 = Enqueue Element(queue=w347, element=w346) -> ()  [unwired: 2 in, 3 out]
          }
          frame True {
          }
        }
      }
      event "move2com": Value Change {
        n180 = event-data() -> ()  [unwired: 1 in, 1 out]
        n181 = Enqueue Element(queue=w349, element="mov2cursor") -> ()  [unwired: 2 in, 3 out]
      }
      event "showcom": Value Change {
        n182 = event-data() -> ()  [unwired: 1 in, 1 out]
        n183 = Enqueue Element(queue=w351, element="showcom") -> ()  [unwired: 2 in, 3 out]
      }
      event "volt_set": Value Change {
        n184 = event-data() -> ()  [unwired: 1 in, 1 out]
        n185 = Number To Fractional String(number="Nominal Voltage") -> (F-format string=w352:string)  [unwired: 3 in]
        n186 = Concatenate Strings("set:" ("element"), w352) -> (w355:string)
        n187 = Enqueue Element(queue=w356, element=w355) -> ()  [unwired: 2 in, 3 out]
      }
    }
  }
  n188 = while {
    tunnel: w40 -> [w375]
    shift-right: [w373] -> _
    shift-left: _ -> [w372]
    shift-right: [w371] -> _
    shift-left: _ -> [w370]
    shift-right: [w369] -> _
    shift-left: _ -> [w368]
    shift-right: [w367] -> _
    shift-left: _ -> [w366]
    shift-right: [w364] -> _
    shift-left: -1 -> [w365]
    tunnel: w41 -> [w363]
    tunnel: w32 -> [w362]
    shift-right: [w361] -> _
    shift-left: _ -> [w360]
    shift-right: [w358] -> _
    shift-left: _ -> [w359]
    stop <- w374 stop-if-true
    # "HAMAMATSU"
    n189 = Preview Queue Element(queue=w375, timeout in ms (-1)=w365) -> (element=w379:string)  [unwired: 1 in, 3 out]
    n190 = Match Pattern(string=w379, regular expression=":") -> (before substring=w377:string, after substring=w376:string)  [unwired: 1 in, 2 out]
    n191 = case shown="\"set\"" w377 {
      tunnel: w376 -> [_ _ w485 _ _ w575 _ _ _ _]
      tunnel: w375 -> [_ w418 w486 w520 w569 w579 w591 w594 w620 w642]
      tunnel: [_ _ _ _ _ _ _ _ _ TRUE] -> w374
      tunnel: [w398 w420 w489 w525 w567 w576 w583 w599 w608 w637] -> w373
      tunnel: w372 -> [w400 w423 w491 w527 w567 w576 w587 _ w634 w637]
      tunnel: [w399 w415 w490 w524 w566 w577 u32 0 ("Handle out") w597 w609 w638] -> w371
      tunnel: w370 -> [w401 w421 w492 w528 w566 w577 w588 _ w632 w638]
      tunnel: [w397 w422 w484 w523 w568 w578 w589 w595 w621 w639] -> w369
      tunnel: w368 -> [w397 w422 w484 w523 w568 w578 w589 w595 _ w639]
      tunnel: [w396 w419 w493 w526 w565 w572 w590 w596 w612 w640] -> w367
      tunnel: w366 -> [w396 w419 w493 w526 _ _ w590 w596 w612 w640]
      tunnel: [0 _ _ _ _ _ _ _ _ _] -> w364
      tunnel: w363 -> [_ w414 w494 _ _ _ _ _ _ _]
      tunnel: w362 -> [_ _ _ w521 _ _ _ _ _ _]
      tunnel: [w382 w409 w488 w512 w564 w571 w581 w593 w614 w636] -> w361
      tunnel: w360 -> [w391 w412 w488 w515 w564 w571 w581 w593 w614 w636]
      tunnel: w359 -> [w386 w411 w487 w513 w563 w570 w580 w592 w613 w635]
      tunnel: [w385 w408 w487 w511 w563 w570 w580 w592 w613 w635] -> w358
      tunnel: "array size" -> [w384 w410 _ w514 _ _ _ _ _ _]
      frame "idle", Default {
        n192 = local read "threshold"() -> (w402:i32)
        n193 = call "tm_getnextframe_a.vi"("error in (no error)"=w400, "Buffer"=w397, "Handle in"=w401) -> ("error out"=w398:errorcluster, "Data"=w392:u16[][], "Handle out"=w399:u32)  [unwired: 6 in]
        n194 = local read "dark?"() -> (w403:bool)
        n195 = local read "count?"() -> (w393:bool)
        n196 = case shown="False" w403 {
          tunnel: [w404 w407] -> w394
          tunnel: w392 -> [w404 w406]
          tunnel: w396 -> [_ w405]
          frame False {
          }
          frame True {
            n197 = Subtract(x=w406, y=w405) -> (x-y=w407:dbl[][])
          }
        }
        n198 = call "filtr_b.vi"("count?"=w393, "threshold"=w402, "input array"=w394) -> ("output array"=w380:dbl[][])  [unwired: 8 in]
        n199 = Add Array Elements(numeric array=w380) -> (sum=w381:dbl)
        n200 = call "ringbuffer.vi"("new val"=w381, "index in"=w386, "array size"=w384, "array in"=w391) -> ("index out"=w385:i32, "array out"=w382:dbl[])  [unwired: 6 in]
        n201 = local write "live"(w380) -> ()
        n202 = local write "Waveform Chart"(w381) -> ()
        n203 = call <vilib>:"Std Deviation and Variance.vi"("X"=w382) -> ("mean"=w387:dbl, "standard deviation"=w390:dbl)  [unwired: 1 in, 1 out]
        n204 = Divide(x=w390, y=w387) -> (x/y=w389:dbl)
        n205 = Multiply(x=w389, y=100.0) -> (x*y=w383:dbl)
        n206 = local write "noise-o-meter"(w383) -> ()
      }
      frame "snap" {
        n207 = Dequeue Element(queue=w418) -> ()  [unwired: 2 in, 4 out]
        n208 = local read "avg[t] acc[f]"() -> (w417:bool)
        n209 = local read "threshold"() -> (w425:i32)
        n210 = local read "frames"() -> (w424:i32)
        n211 = local read "count?"() -> (w416:bool)
        n212 = local read "dark?"() -> (w426:bool)
        n213 = for {
          N: w424 -> [w450]
          tunnel: w426 -> [w464]
          tunnel: w422 -> [w462]
          tunnel: w421 -> [w463]
          tunnel: w425 -> [w456]
          tunnel: [w460] -> w415
          shift-right: [w459] -> w420
          shift-left: w423 -> [w461]
          tunnel: w419 -> [w455]
          shift-right: [w431] -> w413
          shift-left: w422 -> [w453]
          tunnel: w417 -> [w454]
          tunnel: w416 -> [w452]
          shift-right: [w443] -> w409
          shift-left: w412 -> [w444]
          tunnel: w410 -> [w441]
          shift-right: [w440] -> w408
          shift-left: w411 -> [w442]
          shift-right: [w436] -> _
          shift-left: _ -> [w437]
          i -> [w451]
          stop <- "stop" stop-if-true
          n214 = call "tm_getnextframe_a.vi"("error in (no error)"=w461, "Buffer"=w462, "Handle in"=w463) -> ("error out"=w459:errorcluster, "Data"=w458:u16[][], "Handle out"=w460:u32)  [unwired: 6 in]
          n215 = Divide(x=w451, y=w450) -> (x/y=w449:dbl)
          n216 = case shown="True" w464 {
            tunnel: [w475 w478] -> w457
            tunnel: w458 -> [w475 w477]
            tunnel: w455 -> [_ w476]
            frame False {
            }
            frame True {
              n217 = Subtract(x=w477, y=w476) -> (x-y=w478:dbl[][])
            }
          }
          n218 = local write "Slide"(w449) -> ()
          n219 = Tick Count (ms)() -> (millisecond timer value=w436:u32)
          n220 = call "filtr_b.vi"("count?"=w452, "threshold"=w456, "input array"=w457) -> ("output array"=w433:dbl[][])  [unwired: 8 in]
          n221 = Subtract(x=w436, y=w437) -> ()  [unwired: 1 out]
          n222 = Add Array Elements(numeric array=w433) -> (sum=w432:dbl)
          n223 = call "ringbuffer.vi"("new val"=w432, "index in"=w442, "array size"=w441, "array in"=w444) -> ("index out"=w440:i32, "array out"=w443:dbl[])  [unwired: 6 in]
          n224 = call <vilib>:"Std Deviation and Variance.vi"("X"=w443) -> ("mean"=w445:dbl, "standard deviation"=w447:dbl)  [unwired: 1 in, 1 out]
          n225 = local write "live"(w433) -> ()
          n226 = local write "Waveform Chart"(w432) -> ()
          n227 = Divide(x=w447, y=w445) -> (x/y=w439:dbl)
          n228 = case shown="True" w454 {
            tunnel: w453 -> [w467 w474]
            tunnel: w433 -> [w466 w472]
            tunnel: [w465 w468] -> w431
            tunnel: w451 -> [_ w469]
            frame False {
              n229 = Add(x=w467, y=w466) -> (x+y=w465:dbl[][])
            }
            frame True {
              n230 = Multiply(x=w474, y=w469) -> (x*y=w473:dbl[][])
              n231 = Increment(x=w469) -> (x+1=w470:i32)
              n232 = Add(x=w473, y=w472) -> (x+y=w471:dbl[][])
              n233 = Divide(x=w471, y=w470) -> (x/y=w468:dbl[][])
            }
          }
          n234 = local write "captured"(w431) -> ()
          n235 = Multiply(x=w439, y=100.0) -> (x*y=w438:dbl)
          n236 = local write "noise-o-meter"(w438) -> ()
          n237 = Array Size(array=w433) -> (size(s)=w435:i32[])
          n238 = Multiply Array Elements(1:w435) -> (0:w434:i32)
          n239 = local read "stats"() -> (w429:dbl)
          n240 = Add Array Elements(numeric array=w431) -> (sum=w430:dbl)
          n241 = Divide(x=w430, y=w434) -> (x/y=w428:dbl)
          n242 = Divide(x=w429, y=w428) -> (x/y=w427:dbl)
          n243 = local write "x*y"(w427) -> ()
        }
        n244 = local write "captured"(w413) -> ()
        n245 = Enqueue Element(queue=w414, element=w413) -> ()  [unwired: 2 in, 3 out]
      }
      frame "single" {
        n246 = Dequeue Element(queue=w486) -> ()  [unwired: 2 in, 4 out]
        n247 = Decimal String To Number(string=w485) -> (number=w480:i32)  [unwired: 2 in, 1 out]
        n248 = To Unsigned Quad Integer(1:w484) -> (0:w483:u64[][])
        n249 = for {
          N: w480 -> [_]
          tunnel: w484 -> [w506]
          tunnel: w492 -> [w505]
          tunnel: w491 -> [w504]
          tunnel: [w503] -> w490
          tunnel: [w502] -> w489
          shift-right: [w499] -> w482
          shift-left: w483 -> [w501]
          n250 = call "tm_getnextframe_a.vi"("error in (no error)"=w504, "Buffer"=w506, "Handle in"=w505) -> ("error out"=w502:errorcluster, "Data"=w500:u16[][], "Handle out"=w503:u32)  [unwired: 6 in]
          n251 = Add(x=w500, y=w501) -> (x+y=w499:u64[][])
        }
        n252 = local read "dark?"() -> (w495:bool)
        n253 = Divide(x=w482, y=w480) -> (x/y=w481:dbl[][])
        n254 = case shown="True" w495 {
          tunnel: [w507 w510] -> w498
          tunnel: w481 -> [w507 w509]
          tunnel: w493 -> [_ w508]
          frame False {
          }
          frame True {
            n255 = Subtract(x=w509, y=w508) -> (x-y=w510:dbl[][])
          }
        }
        n256 = local read "threshold"() -> (w496:i32)
        n257 = local read "count?"() -> (w497:bool)
        n258 = call "filtr_b.vi"("count?"=w497, "threshold"=w496, "input array"=w498) -> ("output array"=w479:dbl[][])  [unwired: 8 in]
        n259 = Enqueue Element(queue=w494, element=w479) -> ()  [unwired: 2 in, 3 out]
        n260 = local write "captured"(w479) -> ()
      }
      frame "snap_I" {
        n261 = Dequeue Element(queue=w520) -> ()  [unwired: 2 in, 4 out]
        n262 = local read "threshold"() -> (w531:i32)
        n263 = local read "frames"() -> (w530:i32)
        n264 = local read "count?"() -> (w529:bool)
        n265 = local read "dark?"() -> (w532:bool)
        n266 = for {
          N: w530 -> [w546]
          tunnel: w532 -> [w558]
          tunnel: w523 -> [w556]
          tunnel: w528 -> [w557]
          tunnel: w531 -> [w550]
          tunnel: [w554] -> w524
          shift-right: [w553] -> w525
          shift-left: w527 -> [w555]
          tunnel: w526 -> [w549]
          tunnel: w529 -> [w548]
          tunnel: [w544] -> w522 mode=indexing
          shift-right: [w536] -> w512
          shift-left: w515 -> [w537]
          tunnel: w514 -> [w535]
          shift-right: [w533] -> w511
          shift-left: w513 -> [w534]
          i -> [w547]
          n267 = call "tm_getnextframe_a.vi"("error in (no error)"=w555, "Buffer"=w556, "Handle in"=w557) -> ("error out"=w553:errorcluster, "Data"=w552:u16[][], "Handle out"=w554:u32)  [unwired: 6 in]
          n268 = call "ringbuffer.vi"("index in"=w534, "array size"=w535, "array in"=w537) -> ("index out"=w533:i32, "array out"=w536:dbl[])  [unwired: 7 in]
          n269 = Divide(x=w547, y=w546) -> (x/y=w545:dbl)
          n270 = case shown="True" w558 {
            tunnel: [w559 w562] -> w551
            tunnel: w552 -> [w559 w561]
            tunnel: w549 -> [_ w560]
            frame False {
            }
            frame True {
              n271 = Subtract(x=w561, y=w560) -> (x-y=w562:dbl[][])
            }
          }
          n272 = local write "Slide"(w545) -> ()
          n273 = call <vilib>:"Std Deviation and Variance.vi"("X"=w536) -> ("mean"=w538:dbl, "standard deviation"=w541:dbl)  [unwired: 1 in, 1 out]
          n274 = call "filtr_b.vi"("count?"=w548, "threshold"=w550, "input array"=w551) -> ("output array"=w543:dbl[][])  [unwired: 8 in]
          n275 = Divide(x=w541, y=w538) -> (x/y=w540:dbl)
          n276 = local write "live"(w543) -> ()
          n277 = Multiply(x=w540, y=100.0) -> (x*y=w542:dbl)
          n278 = local write "noise-o-meter"(w542) -> ()
          n279 = Add Array Elements(numeric array=w543) -> (sum=w544:dbl)
          n280 = local write "Waveform Chart"(w544) -> ()
        }
        n281 = call <vilib>:"Std Deviation and Variance.vi"("X"=w522) -> ("mean"=w519:dbl, "standard deviation"=w518:dbl)  [unwired: 1 in, 1 out]
        n282 = Format Into String(format string="%.6e;%.6e", w519, w518) -> (resulting string=w517:string)  [unwired: 2 in, 1 out]
        n283 = Enqueue Element(queue=w521, element=w517) -> ()  [unwired: 2 in, 3 out]
      }
      frame "dark" {
        n284 = Dequeue Element(queue=w569) -> ()  [unwired: 2 in, 4 out]
        n285 = local read "captured"() -> (w565:dbl[][])
      }
      frame "dark_load" {
        n286 = Dequeue Element(queue=w579) -> ()  [unwired: 2 in, 4 out]
        n287 = String To Path(string=w575) -> (path=w574:path)
        n288 = Read from Binary File(5:dbl[][] [] ("all rows"), 11:w574) -> (2:w572:dbl[][])  [unwired: 4 in, 3 out]
        n289 = call-poly <vilib>:"Read From Spreadsheet File.vi"("file path (dialog if empty)"=w574) -> ()  [unwired: 6 in, 5 out]
      }
      frame "release" {
        n290 = call "tm_stopcapture.vi"("error in (no error)"=w587, "Handle in"=w588) -> ("error out"=w585:errorcluster, "Handle out"=w586:u32)  [unwired: 8 in]
        n291 = Dequeue Element(queue=w591) -> ()  [unwired: 2 in, 4 out]
        n292 = call "tm_closecamera.vi"("error in (no error)"=w585, "Handle in"=w586) -> ("error out"=w584:errorcluster)  [unwired: 9 in]
        n293 = call "tm_deinitialize.vi"("error in (no error)"=w584) -> ("error out"=w583:errorcluster)  [unwired: 10 in]
      }
      frame "init" {
        n294 = Dequeue Element(queue=w594) -> ()  [unwired: 2 in, 4 out]
        n295 = call "tm_initialize.vi"() -> ("error out"=w600:errorcluster)  [unwired: 8 in, 3 out]
        n296 = call "tm_opencamera.vi"("error in (no error)"=w600, "Camera Index"=u32 0) -> ("error out"=w599:errorcluster, "Handle out"=w597:u32)  [unwired: 7 in, 1 out]
      }
      frame "set" {
        w626 = 1 items=["Snap", "Sequence"] ("Capture mode")
        w627 = u32 4215968 items=["BINNING"=4215968, "BITS PER CHANNEL"=2, "ACTIVE VIEW INDEX"=3, "CCD MODE"=4, "SENSOR MODE"=5, "READOUT MODE"=6, "EXPOSURE TIME"=7, "CONTRAST GAIN"=8, "CONTRAST OFFSET"=9, "LIGHT MODE"=10, "SENSITIVITY"=11, "WHITE BALANCE"=12, "PHOTON IMAGING MODE"=13, "HIGH DYNAMIC RANGE MODE"=14, "TRIGGER SOURCE"=15, "TRIGGER ACTIVE"=16, "TRIGGER MODE"=17, "TRIGGER POLARITY"=18, "TRIGGER GLOBAL EXPOSURE"=19, "FIRST TRIGGER BEHAVIOR"=20, "TRIGGER TIMES"=21, "OUTPUT TRIGGER POLARITY"=22, "OUTPUT TRIGGER DELAY"=23, "OUTPUT TRIGGER PERIOD"=24, "TEMPERATURE"=25, "TEMPERATURE TARGET"=26, "SENSOR COOLER FAN"=27, "MECHANICAL SHUTTER"=28, "BACK FOCUS POSITION"=29, "FRAMEBUNDLE MODE"=30, "FRAMEBUNDLE NUMBER"=31, "LINEBUNDLE HEIGHT"=32, "TRIGGER CONNECTOR"=33, "IMAGE PIXEL TYPE"=34, "OUTPUT TRIGGER KIND"=35, "READOUT DIRECTION"=36, "CHANNEL SYNC"=37] ("Parameter")
        w604 = u32 7 items=["BINNING"=4215968, "BITS PER CHANNEL"=2, "ACTIVE VIEW INDEX"=3, "CCD MODE"=4, "SENSOR MODE"=5, "READOUT MODE"=6, "EXPOSURE TIME"=7, "CONTRAST GAIN"=8, "CONTRAST OFFSET"=9, "LIGHT MODE"=10, "SENSITIVITY"=11, "WHITE BALANCE"=12, "PHOTON IMAGING MODE"=13, "HIGH DYNAMIC RANGE MODE"=14, "TRIGGER SOURCE"=15, "TRIGGER ACTIVE"=16, "TRIGGER MODE"=17, "TRIGGER POLARITY"=18, "TRIGGER GLOBAL EXPOSURE"=19, "FIRST TRIGGER BEHAVIOR"=20, "TRIGGER TIMES"=21, "OUTPUT TRIGGER POLARITY"=22, "OUTPUT TRIGGER DELAY"=23, "OUTPUT TRIGGER PERIOD"=24, "TEMPERATURE"=25, "TEMPERATURE TARGET"=26, "SENSOR COOLER FAN"=27, "MECHANICAL SHUTTER"=28, "BACK FOCUS POSITION"=29, "FRAMEBUNDLE MODE"=30, "FRAMEBUNDLE NUMBER"=31, "LINEBUNDLE HEIGHT"=32, "TRIGGER CONNECTOR"=33, "IMAGE PIXEL TYPE"=34, "OUTPUT TRIGGER KIND"=35, "READOUT DIRECTION"=36, "CHANNEL SYNC"=37] ("Parameter")
        n297 = Dequeue Element(queue=w620) -> ()  [unwired: 2 in, 4 out]
        n298 = call "tm_stopcapture.vi"("error in (no error)"=w634, "Handle in"=w632) -> ("error out"=w633:errorcluster, "Handle out"=w631:u32)  [unwired: 8 in]
        n299 = call "tm_unpreparecapture.vi"("error in (no error)"=w633, "Handle in"=w631) -> ("error out"=w630:errorcluster, "Handle out"=w629:u32)  [unwired: 8 in]
        n300 = call "tm_setparameter.vi"("error in (no error)"=w630, "Value in"="t_exp", "Parameter"=w604, "Handle in"=w629) -> ("error out"=w606:errorcluster, "Handle out"=w605:u32)  [unwired: 6 in]
        n301 = call "tm_getparameter.vi"("error in (no error)"=w606, "Parameter"=w604, "Handle in"=w605) -> ("error out"=w602:errorcluster, "Value out"=w601:dbl, "Handle out"=w603:u32)  [unwired: 6 in]
        n302 = local write "t_exp"(w601) -> ()
        n303 = call "tm_setparameter.vi"("error in (no error)"=w602, "Value in"="Value in", "Parameter"=w627, "Handle in"=w603) -> ("error out"=w610:errorcluster, "Handle out"=w611:u32)  [unwired: 6 in]
        n304 = call "tm_preparecapture.vi"("error in (no error)"=w610, "Frames"=1, "Capture mode"=w626, "Handle in"=w611) -> ("error out"=w623:errorcluster, "Buffer Info"=w622:T5, "Handle out"=w624:u32)  [unwired: 4 in, 1 out]
        n305 = call "tm_startcapture_b.vi"("error in (no error)"=w623, "Handle in"=w624) -> ("error out"=w608:errorcluster, "Handle out"=w609:u32)  [unwired: 8 in]
        n306 = Unbundle(w622) -> ("height"=w618:u32, "width"=w619:u32)  [unwired: 1 out]
        n307 = property on="live" class="IntGraph (strict)"("XScale.Minimum"=0.0 ("X Scale.Range:Minimum"), "XScale.Maximum"=w618, "YScale.Minimum"=0.0 ("Y Scale.Range:Minimum"), "YScale.Maximum"=w619) -> ()  [unwired: 2 in, 2 out]
        n308 = Initialize Array(u16 0 ("element"), w618, w619) -> (w621:u16[][])
      }
      frame "close" {
        n309 = Release Queue(queue=w642) -> ()  [unwired: 2 in, 3 out]
      }
    }
  }
  n310 = while {
    tunnel: w35 -> [w651]
    shift-right: [w649] -> _
    shift-left: _ -> [w648]
    shift-right: [w646] -> _
    shift-left: -1 -> [w647]
    shift-right: [w645] -> _
    shift-left: _ -> [w644]
    tunnel: w32 -> [w643]
    stop <- w650 stop-if-true
    # "ISEG"
    n311 = Preview Queue Element(queue=w651, timeout in ms (-1)=w647) -> (element=w655:string)  [unwired: 1 in, 3 out]
    n312 = Match Pattern(string=w655, regular expression=":") -> (before substring=w653:string, after substring=w652:string)  [unwired: 1 in, 2 out]
    n313 = case shown="\"idle\", Default" w653 {
      tunnel: w652 -> [_ w671 _ _ _]
      tunnel: w651 -> [_ w683 w725 w729 w733]
      tunnel: [_ _ _ _ TRUE] -> w650
      tunnel: [w660 w677 w723 w728 w730] -> w649
      tunnel: w648 -> [w662 w681 _ _ w730]
      tunnel: [0 _ _ _ _] -> w646
      tunnel: [w661 w678 T6 {"VISA Resource Name"="", "FP Notation"=FALSE, "Maximum Voltage"=0, "Maximum Current"=0} ("VISA Session Out") w726 w731] -> w645
      tunnel: w644 -> [w663 w682 w724 _ w731]
      tunnel: w643 -> [_ w666 _ _ _]
      frame "idle", Default {
        n314 = local read "Channel (A)"() -> (w664:enum16{"A", "B"})
        n315 = call "iseg NHQ xxx GetActualVoltage.vi"("error in (no error)"=w662, "Channel (A)"=w664, "VISA Session"=w663) -> ("error out"=w660:errorcluster, "Voltage"=w658:dbl, "VISA Session Out"=w661:T6)  [unwired: 5 in, 1 out]
        n316 = Round To Nearest(number=w658) -> (nearest integer value=w657:dbl)
        n317 = node(w658) -> (→"Actual Voltage":dbl[unit])
        n318 = Absolute Value(x=w657) -> (abs(x)=w656:dbl)
        n319 = local write "meas_voltage"(w656) -> ()
      }
      frame "set" {
        n320 = local read "Channel (A)"() -> (w674:enum16{"A", "B"})
        n321 = Dequeue Element(queue=w683) -> ()  [unwired: 2 in, 4 out]
        n322 = Match Pattern(string=w671, regular expression=":") -> (before substring=w670:string, after substring=w669:string)  [unwired: 1 in, 2 out]
        n323 = Fract/Exp String To Number(string=w670) -> (number=w673:dbl)  [unwired: 3 in, 1 out]
        n324 = call "iseg NHQ xxx SetNominalVoltage.vi"("error in (no error)"=w681, "Voltage (0 V)"=w673, "Channel (A)"=w674, "VISA Session"=w682) -> ("error out"=w684:errorcluster, "VISA Session Out"=w685:T6)  [unwired: 6 in]
        n325 = Equal?(x=w669, y="wait") -> (x = y?=w667:bool)
        n326 = call "iseg NHQ xxx StartVoltageChange.vi"("error in (no error)"=w684, "Channel (A)"=w674, "VISA Session"=w685) -> ("error out"=w679:errorcluster, "VISA Session Out"=w680:T6)  [unwired: 6 in, 1 out]
        n327 = case shown="True" w667 {
          tunnel: [w687 w697] -> w678
          tunnel: [w686 w689] -> w677
          tunnel: w680 -> [w687 w696]
          tunnel: w679 -> [w686 w695]
          tunnel: w673 -> [_ w694]
          tunnel: "volt_threshold" -> [_ w693]
          tunnel: "volt_timeout" -> [_ w692]
          tunnel: w674 -> [_ w691]
          tunnel: w666 -> [_ w690]
          frame False {
          }
          frame True {
            n328 = Tick Count (ms)() -> (millisecond timer value=w698:u32)
            n329 = while {
              shift-right: [w719] -> w697
              shift-left: w696 -> [w721]
              shift-right: [w706] -> w689
              shift-left: w695 -> [w720]
              tunnel: w691 -> [w718]
              tunnel: w693 -> [w715]
              tunnel: w698 -> [w713]
              tunnel: w692 -> [w711]
              tunnel: w694 -> [w710]
              tunnel: [w701] -> w688
              stop <- w707 stop-if-true
              n330 = Tick Count (ms)() -> (millisecond timer value=w714:u32)
              n331 = call "iseg NHQ xxx GetActualVoltage.vi"("error in (no error)"=w720, "Channel (A)"=w718, "VISA Session"=w721) -> ("error out"=w706:errorcluster, "Voltage"=w699:dbl, "VISA Session Out"=w719:T6)  [unwired: 5 in, 1 out]
              n332 = Absolute Value(x=w699) -> (abs(x)=w709:dbl)
              n333 = node(w699) -> (w700:dbl[unit])
              n334 = Subtract(x=w714, y=w713) -> (x-y=w712:u32)
              n335 = Subtract(x=w709, y=w710) -> (x-y=w717:dbl)
              n336 = local write "Actual Voltage"(w700) -> ()
              n337 = Absolute Value(x=w717) -> (abs(x)=w716:dbl)
              n338 = Greater?(x=w712, y=w711) -> (0:w705:bool)
              n339 = Less?(x=w716, y=w715) -> (x < y?=w708:bool)
              n340 = Or(x=w706, y=w705) -> (x .or. y?=w704:bool)
              n341 = Compound Arithmetic op=OR(w706, w708, w705) -> (w707:bool)
              n342 = Select(t="fail" ("element"), s=w704, f="done" ("element")) -> (s? t:f=w701:string)
            }
            n343 = Enqueue Element(queue=w690, element=w688) -> ()  [unwired: 2 in, 3 out]
          }
        }
      }
      frame "release" {
        n344 = Dequeue Element(queue=w725) -> ()  [unwired: 2 in, 4 out]
        n345 = call "iseg NHQ xxx Close.vi"("VISA session"=w724) -> ("error out"=w723:errorcluster)  [unwired: 14 in]
      }
      frame "init" {
        n346 = Dequeue Element(queue=w729) -> ()  [unwired: 2 in, 4 out]
        n347 = call "iseg NHQ xxx Initialize.vi"("VISA resource name"="VISA ISEG") -> ("VISA Session Out"=w726:T6, "error out"=w728:errorcluster)  [unwired: 13 in]
      }
      frame "close" {
        n348 = Release Queue(queue=w733) -> ()  [unwired: 2 in, 3 out]
      }
    }
    "error out" <- w649
  }
  n349 = while {
    tunnel: w15 -> [w744]
    shift-right: [w736] -> _
    shift-left: errorcluster {"status"=FALSE, "code"=0, "source"=""} ("error constant") -> [w742]
    shift-right: [w738] -> _
    shift-left: _ -> [w734]
    shift-right: [w741] -> _
    shift-left: _ -> [w740]
    tunnel: w32 -> [w739]
    tunnel: w13 -> [w735]
    tunnel: [w735] -> w12
    stop <- w743 stop-if-true
    # "COHERENT"
    n350 = Preview Queue Element(queue=w744, timeout in ms (-1)=w734) -> (element=w748:string)  [unwired: 1 in, 3 out]
    n351 = Match Pattern(string=w748, regular expression=":") -> (before substring=w746:string, after substring=w745:string)  [unwired: 1 in, 2 out]
    n352 = case shown="\"start\"" w746 {
      tunnel: w745 -> [_ _ _ _ _ _]
      tunnel: w744 -> [_ w774 w802 w812 w819 w826]
      tunnel: [_ _ _ _ _ TRUE] -> w743
      tunnel: [w756 w768 w796 w810 w816 w823] -> w736
      tunnel: w742 -> [w758 w771 w798 _ w814 w823]
      tunnel: [0 w761 w795 w807 0 w822] -> w737
      tunnel: [w757 w769 w797 0 ("Meter Index") w817 w824] -> w741
      tunnel: w740 -> [w759 w772 w799 w808 _ w824]
      tunnel: w739 -> [_ w770 w801 _ _ _]
      tunnel: w734 -> [_ w761 w795 w807 _ w822]
      frame "idle", Default {
        n353 = call "CH_LM Measurement Fetch Data.vi"("Meter Index"=w759, "error in (no error)"=w758) -> ("Meter Index"=w757:i32, "Data Array"=w755:T7[], "error out"=w756:errorcluster)  [unwired: 13 in, 2 out]
        n354 = Index Array(array=w755) -> (element=w754:T7)  [unwired: 1 in]
        n355 = Unbundle By Name(w754) -> ("Value"=w753:sgl)
        n356 = local read "x"() -> (w752:sgl)
        n357 = Multiply(x=w752, y=w753) -> (x*y=→"laser power" →"meas_power":sgl)
      }
      frame "start" {
        n358 = Dequeue Element(queue=w774) -> (queue out=w773:refnum<queue>)  [unwired: 2 in, 3 out]
        n359 = while {
          tunnel: w773 -> [w788]
          tunnel: w772 -> [w785]
          tunnel: w771 -> [w784]
          tunnel: [w783] -> w769
          tunnel: [w782] -> w768
          shift-right: [w779] -> w762
          shift-left: dbl[] [] -> [w780]
          stop <- w789 continue-if-true
          n360 = call "CH_LM Measurement Fetch Data.vi"("Meter Index"=w785, "error in (no error)"=w784) -> ("Meter Index"=w783:i32, "Data Array"=w787:T7[], "error out"=w782:errorcluster)  [unwired: 13 in, 2 out]
          n361 = Index Array(array=w787) -> (element=w786:T7)  [unwired: 1 in]
          n362 = Dequeue Element(queue=w788, timeout in ms (-1)=0) -> (element=w791:string)  [unwired: 1 in, 3 out]
          n363 = Equal?(x=w791, y="") -> (x = y?=w789:bool)
          n364 = Unbundle By Name(w786) -> ("Value"=w776:sgl)
          n365 = local read "x"() -> (w777:sgl)
          n366 = Multiply(x=w777, y=w776) -> (x*y=w775:sgl)
          n367 = Build Array (concatenate)(w780, w775) -> (w779:dbl[])
          n368 = local write "laser power"(w775) -> ()
          n369 = call <vilib>:"Std Deviation and Variance.vi"("X"=w779) -> ("mean"=w778:dbl)  [unwired: 1 in, 2 out]
          n370 = local write "meas_power"(w778) -> ()
        }
        n371 = call <vilib>:"Std Deviation and Variance.vi"("X"=w762) -> ("mean"=w764:dbl, "standard deviation"=w766:dbl)  [unwired: 1 in, 1 out]
        n372 = Format Into String(format string="%.6e;%.6e", w764, w766) -> (resulting string=w765:string)  [unwired: 2 in, 1 out]
        n373 = Enqueue Element(queue=w770, element=w765) -> ()  [unwired: 2 in, 3 out]
      }
      frame "snap" {
        n374 = Dequeue Element(queue=w802) -> ()  [unwired: 2 in, 4 out]
        n375 = call "CH_LM Measurement Fetch Data.vi"("Meter Index"=w799, "error in (no error)"=w798) -> ("Meter Index"=w797:i32, "Data Array"=w804:T7[], "error out"=w796:errorcluster)  [unwired: 13 in, 2 out]
        n376 = Index Array(array=w804) -> (element=w803:T7)  [unwired: 1 in]
        n377 = Unbundle By Name(w803) -> ("Value"=w793:sgl)
        n378 = local read "x"() -> (w794:sgl)
        n379 = Multiply(x=w794, y=w793) -> (x*y=w792:sgl)
        n380 = local write "laser power"(w792) -> ()
        n381 = Format Into String(format string="%.6e", w792) -> (resulting string=w800:string)  [unwired: 2 in, 1 out]
        n382 = Enqueue Element(queue=w801, element=w800) -> ()  [unwired: 2 in, 3 out]
      }
      frame "release" {
        n383 = Dequeue Element(queue=w812) -> ()  [unwired: 2 in, 4 out]
        n384 = call "CH_LM Measurement Abort.vi"("Meter Index"=w808) -> ("Meter Index"=w809:i32, "error out"=w806:errorcluster)  [unwired: 16 in, 1 out]
        n385 = call "CH_LM Close.vi"("Meter Index"=w809, "error in (no error)"=w806) -> ("error out"=w810:errorcluster)  [unwired: 15 in, 2 out]
      }
      frame "init" {
        n386 = Dequeue Element(queue=w819) -> ()  [unwired: 2 in, 4 out]
        n387 = flat-sequence {
          tunnel: w814 -> [w820]
          tunnel: [w820] -> w813
          frame #0 {
            n388 = Wait (ms)(milliseconds to wait=u32 10000) -> ()  [unwired: 1 out]
          }
        }
        n389 = call "CH_LM Measurement Initiate.vi"("Meter Index"=0, "error in (no error)"=w813) -> ("Meter Index"=w817:i32, "error out"=w816:errorcluster)  [unwired: 15 in, 1 out]
      }
      frame "close" {
        n390 = Release Queue(queue=w826) -> ()  [unwired: 2 in, 3 out]
      }
    }
    "coherent" <- w736
    n391 = case shown="No Error" w736 {
      tunnel: [w749 -1] -> w738
      tunnel: w737 -> [w749 _]
      frame No Error {
      }
      frame Error {
      }
    }
  }
  n392 = while {
    shift-right: [w829] -> _
    shift-left: _ -> [w837]
    shift-right: [w835] -> _
    shift-left: 200 -> [w836]
    shift-right: [w833] -> _
    shift-left: _ -> [w832]
    tunnel: w29 -> [w830]
    tunnel: w26 -> [w827]
    stop <- w838 stop-if-true
    # "ESP301"
    n393 = Preview Queue Element(queue=w827, timeout in ms (-1)=w836) -> (queue out=w834:refnum<queue>, element=w842:string)  [unwired: 1 in, 2 out]
    n394 = Match Pattern(string=w842, regular expression=":") -> (before substring=w840:string, after substring=w839:string)  [unwired: 1 in, 2 out]
    n395 = case shown="\"idle\", Default" w840 {
      tunnel: w839 -> [_ w868 w908 _ _ _]
      tunnel: [_ _ _ _ _ TRUE] -> w838
      tunnel: [w852 w863 w904 w911 w919 w924] -> w829
      tunnel: w837 -> [w855 w872 w906 w913 _ w924]
      tunnel: w834 -> [_ w859 w900 w910 w920 w922]
      tunnel: [w853 w856 w905 refnum<visa-resource-name> refnum ("VISA resource name out") w918 w923] -> w833
      tunnel: w832 -> [w854 w871 w907 w914 _ w923]
      tunnel: "esp_axis" -> [w851 w857 w903 _ _ _]
      tunnel: w830 -> [_ w861 _ _ _ _]
      tunnel: [200 0 0 0 0 0] -> w828
      frame "idle", Default {
        n396 = call "Read Actual Position.vi"("error in (no error)"=w855, "Axis (1)"=w851, "VISA resource name"=w854) -> ("error out"=w852:errorcluster, "Position (units)"=w846:dbl, "VISA resource name out"=w853:refnum<visa-resource-name>)  [unwired: 2 in]
        "[mm]" <- w846
        n397 = local read "t0 @"() -> (w849:dbl)
        n398 = call "mm2time.vi"("fs?"=TRUE, "Offset (mm)"=w849, "distance (mm)"=w846) -> ("time in fs/ps seconds"=w847:dbl)
        n399 = Negate(x=w847) -> (-x=→"esp_pos_fs":dbl)
      }
      frame "abs" {
        n400 = Dequeue Element(queue=w859) -> ()  [unwired: 2 in, 4 out]
        n401 = Match Pattern(string=w868, regular expression=":") -> (before substring=w867:string, after substring=w866:string)  [unwired: 1 in, 2 out]
        n402 = Equal?(x=w866, y="confirm") -> (x = y?=w862:bool)
        n403 = Fract/Exp String To Number(string=w867) -> (number=w870:dbl)  [unwired: 3 in, 1 out]
        n404 = call "Move Absolute.vi"("error in (no error)"=w872, "Position (0 units)"=w870, "Axis (1)"=w857, "VISA resource name"=w871) -> ("error out"=w864:errorcluster, "VISA resource name out"=w858:refnum<visa-resource-name>)  [unwired: 2 in]
        n405 = case shown="True" w862 {
          tunnel: w864 -> [w874 w879]
          tunnel: [w874 w882] -> w863
          tunnel: w861 -> [_ w881]
          tunnel: w858 -> [w873 w877]
          tunnel: w857 -> [_ w876]
          tunnel: [w873 w875] -> w856
          frame False {
          }
          frame True {
            n406 = while {
              tunnel: w877 -> [w887]
              tunnel: w876 -> [w883]
              shift-right: [w891] -> w878
              shift-left: w879 -> [w886]
              tunnel: [w890] -> w875
              stop <- w893 continue-if-true
              n407 = call "Read Actual Position.vi"("error in (no error)"=w886, "Axis (1)"=w883, "VISA resource name"=w887) -> ("error out"=w884:errorcluster, "Position (units)"=w888:dbl, "VISA resource name out"=w885:refnum<visa-resource-name>)  [unwired: 2 in]
              n408 = local write "[mm]"(w888) -> ()
              n409 = Decrement(x=w883) -> (x-1=w889:i32)
              n410 = call "Get Controller Status.vi"("error in (no error)"=w884, "VISA resource name"=w885) -> ("error out"=w891:errorcluster, "Controller Status"=w899:T8, "VISA resource name out"=w890:refnum<visa-resource-name>)  [unwired: 2 in, 1 out]
              n411 = Unbundle(w899) -> ("Axis1 moving"=w898:bool, "Axis2 moving"=w897:bool, "Axis3 moving"=w896:bool, "Axis4 moving"=w895:bool)  [unwired: 12 out]
              n412 = Build Array(w898, w897, w896, w895) -> (w894:bool[])
              n413 = Index Array(array=w894, index=w889) -> (element=w892:bool)
              n414 = Or(x=w892, y=w891) -> (x .or. y?=w893:bool)
            }
            n415 = Send Notification(notification=TRUE, notifier=w881, error in (no error)=w878) -> (error out=w882:errorcluster)  [unwired: 1 out]
          }
        }
      }
      frame "rel" {
        n416 = Dequeue Element(queue=w900) -> ()  [unwired: 2 in, 4 out]
        n417 = Fract/Exp String To Number(string=w908) -> (number=w902:dbl)  [unwired: 3 in, 1 out]
        n418 = call "Move Relative.vi"("error in (no error)"=w906, "Position (0 units)"=w902, "Axis (1)"=w903, "VISA resource name"=w907) -> ("error out"=w904:errorcluster, "VISA resource name out"=w905:refnum<visa-resource-name>)  [unwired: 2 in]
      }
      frame "release" {
        n419 = Dequeue Element(queue=w910) -> ()  [unwired: 2 in, 4 out]
        n420 = call "Close.vi"("error in (no error)"=w913, "VISA resource name"=w914) -> ("error out"=w911:errorcluster)  [unwired: 9 in]
      }
      frame "init" {
        n421 = Dequeue Element(queue=w920) -> ()  [unwired: 2 in, 4 out]
        n422 = call "Initialize.vi"("VISA resource name"="esp_visa", "Serial Link (RS232)"=enum16{"RS232", "USB"}."RS232") -> ("VISA resource name out"=w918:refnum<visa-resource-name>, "error out"=w919:errorcluster)  [unwired: 7 in]
      }
      frame "close" {
        n423 = Release Queue(queue=w922) -> ()  [unwired: 2 in, 3 out]
      }
    }
    "esp301" <- w829
    n424 = case shown="No Error" w829 {
      tunnel: [w843 -1] -> w835
      tunnel: w828 -> [w843 _]
      frame No Error {
      }
      frame Error {
      }
    }
  }
  n425 = while {
    tunnel: w32 -> [w935]
    tunnel: w41 -> [w934]
    tunnel: w40 -> [w932]
    tunnel: w35 -> [w931]
    tunnel: w15 -> [w930]
    tunnel: w29 -> [w929]
    tunnel: w26 -> [w928]
    tunnel: w3 -> [w927]
    tunnel: w2 -> [w926]
    stop <- w933 stop-if-true
    # "coherent"
    n426 = Preview Queue Element(queue=w935) -> (element=w939:string)  [unwired: 2 in, 3 out]
    n427 = Match Pattern(string=w939, regular expression=":") -> (before substring=w937:string, after substring=w936:string)  [unwired: 1 in, 2 out]
    n428 = case shown="\"power2\"" w937 {
      tunnel: w936 -> [_ _ _ _ _ _ _ _ _ _]
      tunnel: w935 -> [w942 w946 w991 w1057 w1058 w1076 w1206 w1223 w1332 _]
      tunnel: w934 -> [w943 _ w987 _ _ w1068 w1205 w1221 w1330 _]
      tunnel: [TRUE _ _ _ _ _ _ _ _ _] -> w933
      tunnel: w932 -> [_ w945 w988 _ _ w1069 w1204 w1222 w1329 _]
      tunnel: w931 -> [_ _ _ _ _ w1070 w1203 w1220 _ _]
      tunnel: w930 -> [_ _ _ _ _ w1071 w1202 w1219 _ _]
      tunnel: w929 -> [_ _ _ _ _ _ _ _ w1346 _]
      tunnel: w928 -> [_ _ _ _ _ _ _ _ w1327 _]
      tunnel: w927 -> [w940 _ _ _ _ _ w1161 w1215 _ _]
      tunnel: w926 -> [_ _ _ _ _ _ w1162 w1216 _ _]
      frame "close" {
        n429 = Release Queue(queue=w942) -> ()  [unwired: 2 in, 3 out]
        n430 = Release Queue(queue=w943) -> ()  [unwired: 2 in, 3 out]
        n431 = Release Queue(queue=w940) -> ()  [unwired: 2 in, 3 out]
      }
      frame "single" {
        n432 = Dequeue Element(queue=w946) -> ()  [unwired: 2 in, 4 out]
        n433 = Enqueue Element(queue=w945, element="snap") -> ()  [unwired: 2 in, 3 out]
      }
      frame "XY" {
        n434 = local read "IP address"() -> (w947:string)
        n435 = Dequeue Element(queue=w991) -> ()  [unwired: 2 in, 4 out]
        n436 = local read "Path"() -> (w982:path)
        n437 = Get Date/Time In Seconds() -> (seconds since 1Jan1904=w986:timestamp)
        n438 = Format Date/Time String(time format string (%c)="2AxisScan_%Y%m%d_%H%M%S\\raw\\", seconds (now)=w986) -> (date/time string=w951:string)  [unwired: 1 in]
        n439 = Build Path(base path=w982, name or relative path=w951) -> (appended path=w955:path)
        n440 = call "tcp_getpos.vi"("Axis"="Axis1", "IP address"=w947) -> ("error out"=w983:errorcluster, "position"=w960:dbl, "IP address out"=w984:string)  [unwired: 7 in]
        n441 = Concatenate Strings("rows_" ("string"), "Axis1") -> (w952:string)
        n442 = Concatenate Strings("cols_" ("string"), "Axis2") -> (w981:string)
        n443 = Add(x="window1", y=w960) -> (x+y=w967:dbl)
        n444 = Subtract(x=w960, y="window1") -> (x-y=w966:dbl)
        n445 = Create Folder(path (use dialog)=w955) -> (created path=w950:path)  [unwired: 2 in, 2 out]
        n446 = call "tcp_getpos.vi"("error in (no error)"=w983, "Axis"="Axis2", "IP address"=w984) -> ("error out"=w976:errorcluster, "position"=w961:dbl, "IP address out"=w971:string)  [unwired: 6 in]
        n447 = Build Path(base path=w950, name or relative path=w952) -> (appended path=w949:path)
        n448 = Build Path(base path=w950, name or relative path=w981) -> (appended path=w948:path)
        n449 = Add(x="window2", y=w961) -> (x+y=w964:dbl)
        n450 = Subtract(x=w961, y="window2") -> (x-y=w965:dbl)
        n451 = call-poly <vilib>:"Ramp Pattern.vi"("start"=w966, "end"=w967, "samples"="steps1") -> ("Ramp Pattern"=w963:dbl[])  [unwired: 7 in, 1 out]
        n452 = call-poly <vilib>:"Ramp Pattern.vi"("start"=w965, "end"=w964, "samples"="steps2") -> ("Ramp Pattern"=w962:dbl[])  [unwired: 7 in, 1 out]
        n453 = Build Path(base path=w950, name or relative path="intensities") -> (appended path=w953:path)
        n454 = Add(x=w961, y=w963) -> (x+y=w959:dbl[])
        n455 = Add(x=w960, y=w962) -> (x+y=w958:dbl[])
        n456 = Initialize Array(0.0 ("element"), "steps1", "steps2") -> (w989:dbl[][])
        n457 = call-poly <vilib>:"Write To Spreadsheet File.vi"("1D data"=w959, "file path (dialog if empty)"=w949) -> ()  [unwired: 6 in, 1 out]
        n458 = call-poly <vilib>:"Write To Spreadsheet File.vi"("1D data"=w958, "file path (dialog if empty)"=w948) -> ()  [unwired: 6 in, 1 out]
        n459 = for {
          tunnel: "Axis1" -> [w1008]
          tunnel: w988 -> [w1007]
          tunnel: w987 -> [w1006]
          tunnel: "Axis2" -> [w1002]
          shift-right: [w1001] -> w980
          shift-left: w989 -> [w1005]
          shift-right: [w998] -> w977
          shift-left: w976 -> [w997]
          tunnel: [w995] -> w972
          tunnel: w971 -> [w994]
          tunnel: w963 -> [w992] mode=indexing
          tunnel: w962 -> [w993]
          i -> [w1004]
          stop <- w996 stop-if-true
          w1003 = TRUE ("wait4motiondone")
          n460 = call "tcp_move_abs.vi"("wait4motiondone"=w1003, "error in (no error)"=w997, "destination nm/u°"=w992, "Axis"=w1008, "IP address"=w994) -> ("error out"=w1000:errorcluster, "IP address out"=w999:string)  [unwired: 4 in, 1 out]
          n461 = for {
            tunnel: w1007 -> [w1025]
            tunnel: w1006 -> [w1024]
            tunnel: w1004 -> [w1010]
            shift-right: [w1015] -> w1001
            shift-left: w1005 -> [w1023]
            tunnel: w1003 -> [w1019]
            tunnel: w1002 -> [w1018]
            tunnel: w999 -> [w1016]
            shift-right: [w1014] -> w998
            shift-left: w1000 -> [w1017]
            tunnel: ["meas_stop_XY"] -> w996
            tunnel: [w1012] -> w995
            tunnel: w993 -> [w1011] mode=indexing
            i -> [w1009]
            stop <- "meas_stop_XY" stop-if-true
            n462 = call "tcp_move_abs.vi"("wait4motiondone"=w1019, "error in (no error)"=w1017, "destination nm/u°"=w1011, "Axis"=w1018, "IP address"=w1016) -> ("error out"=w1020:errorcluster, "IP address out"=w1012:string)  [unwired: 4 in, 1 out]
            n463 = Enqueue Element(queue=w1025, element="snap", error in (no error)=w1020) -> (error out=w1026:errorcluster)  [unwired: 1 in, 2 out]
            n464 = Dequeue Element(queue=w1024, error in (no error)=w1026) -> (element=w1022:dbl[][], error out=w1014:errorcluster)  [unwired: 1 in, 2 out]
            n465 = Add Array Elements(numeric array=w1022) -> (sum=w1021:dbl)
            n466 = Replace Array Subset(array=w1023, new element=w1021, index (row)=w1010, index (col)=w1009) -> (w1015:dbl[][])
            n467 = local write "XY"(w1015) -> ()
          }
        }
        "XY" <- w980
        n468 = call "tcp_move_abs.vi"("error in (no error)"=w977, "destination nm/u°"=w960, "Axis"="Axis1", "IP address"=w972) -> ("error out"=w979:errorcluster, "IP address out"=w978:string)  [unwired: 5 in, 1 out]
        n469 = call "tcp_move_abs.vi"("error in (no error)"=w979, "destination nm/u°"=w961, "Axis"="Axis2", "IP address"=w978) -> ()  [unwired: 5 in, 3 out]
        n470 = call-poly <vilib>:"Write To Spreadsheet File.vi"("2D data"=w980, "file path (dialog if empty)"=w953) -> ()  [unwired: 6 in, 1 out]
      }
      frame "mov2cursor" {
        n471 = Dequeue Element(queue=w1057) -> ()  [unwired: 2 in, 4 out]
        n472 = local read "IP address"() -> (w1052:string)
        n473 = local read "Axis2"() -> (w1030:string)
        n474 = local read "Axis1"() -> (w1031:string)
        n475 = local read "window1"() -> (w1045:dbl)
        n476 = local read "window2"() -> (w1044:dbl)
        n477 = local read "steps2"() -> (w1050:u32)
        n478 = local read "steps1"() -> (w1051:u32)
        n479 = property on="XY" class="IntGraph (strict)"() -> ("Cursor.Cursor X"=w1029:dbl, "Cursor.Cursor Y"=w1028:dbl)  [unwired: 2 in, 2 out]
        n480 = Multiply(x=2.0, y=w1045) -> (x*y=w1049:dbl)
        n481 = Multiply(x=2.0, y=w1044) -> (x*y=w1046:dbl)
        n482 = Divide(x=w1049, y=w1051) -> (x/y=w1043:dbl)
        n483 = Divide(x=w1046, y=w1050) -> (x/y=w1040:dbl)
        n484 = call "tcp_getpos.vi"("Axis"=w1031, "IP address"=w1052) -> ("error out"=w1055:errorcluster, "position"=w1053:dbl, "IP address out"=w1056:string)  [unwired: 7 in]
        n485 = Subtract(x=w1053, y=w1045) -> (x-y=w1041:dbl)
        n486 = call "tcp_getpos.vi"("error in (no error)"=w1055, "Axis"=w1030, "IP address"=w1056) -> ("error out"=w1033:errorcluster, "position"=w1054:dbl, "IP address out"=w1032:string)  [unwired: 6 in]
        n487 = Subtract(x=w1054, y=w1044) -> (x-y=w1038:dbl)
        n488 = Multiply(x=w1029, y=w1043) -> (x*y=w1042:dbl)
        n489 = Multiply(x=w1028, y=w1040) -> (x*y=w1039:dbl)
        n490 = Add(x=w1041, y=w1042) -> (x+y=w1035:dbl)
        n491 = Add(x=w1039, y=w1038) -> (x+y=w1034:dbl)
        n492 = call "tcp_move_abs.vi"("error in (no error)"=w1033, "destination nm/u°"=w1035, "Axis"=w1031, "IP address"=w1032) -> ("error out"=w1037:errorcluster, "IP address out"=w1036:string)  [unwired: 5 in, 1 out]
        n493 = call "tcp_move_abs.vi"("error in (no error)"=w1037, "destination nm/u°"=w1034, "Axis"=w1030, "IP address"=w1036) -> ()  [unwired: 5 in, 3 out]
      }
      frame "showcom" {
        n494 = Dequeue Element(queue=w1058) -> ()  [unwired: 2 in, 4 out]
        n495 = local read "XY"() -> (w1061:dbl[][])
        n496 = call "COM.vi"("Array"=w1061) -> ("Y out"=w1059:dbl, "X out"=w1060:dbl)  [unwired: 3 in]
        n497 = property on="XY" class="IntGraph (strict)"("Cursor.Cursor X"=w1060, "Cursor.Cursor Y"=w1059) -> ()  [unwired: 2 in, 2 out]
      }
      frame "volt" {
        n498 = Flush Queue(queue=w1076) -> (queue out=w1072:refnum<queue>)  [unwired: 1 in, 2 out]
        n499 = local read "Path"() -> (w1075:path)
        n500 = Build Path(base path=w1075, name or relative path="head") -> (appended path=w1063:path)
        n501 = Build Path(base path=w1063, name or relative path="raw") -> (appended path=w1065:path)
        n502 = Build Path(base path=w1063, name or relative path="LUT.txt") -> (appended path=w1066:path)
        n503 = Create Folder(path (use dialog)=w1065) -> (created path=w1064:path)  [unwired: 2 in, 2 out]
        n504 = while {
          tunnel: w1072 -> [w1077]
          tunnel: w1071 -> [w1100]
          tunnel: w1070 -> [w1094]
          tunnel: w1069 -> [w1093]
          tunnel: w1068 -> [w1092]
          tunnel: w1066 -> [w1087]
          tunnel: w1064 -> [w1086]
          shift-right: [w1079] -> _
          shift-left: _ -> [w1084]
          tunnel: [w1077] -> w1062
          i -> [w1091]
          stop <- w1078 stop-if-true
          n505 = call-poly <vilib>:"Ramp Pattern.vi"("start"="volt_start", "end"="volt_end", "samples"="volt_samples") -> ("Ramp Pattern"=w1090:dbl[])  [unwired: 7 in, 1 out]
          n506 = Array Size(array=w1090) -> (size(s)=w1089:i32)
          n507 = Number To Fractional String(number=w1090) -> (F-format string=w1096:string[])  [unwired: 3 in]
          n508 = Multiply(x=w1089, y=w1091) -> (x*y=w1088:i32)
          n509 = for {
            N -> [w1103]
            tunnel: w1100 -> [w1130]
            tunnel: w1077 -> [w1137]
            tunnel: w1096 -> [w1120] mode=indexing
            tunnel: "set:" ("element") -> [w1134]
            tunnel: w1094 -> [w1133]
            tunnel: w1077 -> [w1131]
            tunnel: w1093 -> [w1128]
            tunnel: w1092 -> [w1125]
            shift-right: [w1105] -> w1085
            shift-left: w1084 -> [w1123]
            tunnel: w1088 -> [w1122]
            tunnel: w1087 -> [w1119]
            tunnel: w1086 -> [w1118]
            tunnel: ":wait" ("element") -> [w1104]
            i -> [w1102]
            n510 = Concatenate Strings(w1134, w1120, w1104) -> (w1135:string)
            n511 = Add(x=w1122, y=w1102) -> (x+y=w1121:i32)
            n512 = Divide(x=w1102, y=w1103) -> (x/y=→"Slide 2":dbl)
            n513 = Number To Decimal String(number=w1121) -> (decimal integer string=w1117:string)  [unwired: 1 in]
            n514 = Enqueue Element(queue=w1133, element=w1135, error in (no error)=w1123) -> (error out=w1132:errorcluster)  [unwired: 1 in, 2 out]
            n515 = Dequeue Element(queue=w1131, error in (no error)=w1132) -> (element=w1114:string, error out=w1112:errorcluster)  [unwired: 1 in, 2 out]
            n516 = Equal?(x="stop" ("y"), y=w1114) -> (x = y?=w1111:bool)
            n517 = call "inject_error.vi"("error in"=w1112, "s"=w1111) -> ("error out"=w1113:errorcluster)  [unwired: 9 in]
            n518 = Enqueue Element(queue=w1130, element="start", error in (no error)=w1113) -> (error out=w1127:errorcluster)  [unwired: 1 in, 2 out]
            n519 = Enqueue Element(queue=w1128, element="snap", error in (no error)=w1127) -> (error out=w1126:errorcluster)  [unwired: 1 in, 2 out]
            n520 = Dequeue Element(queue=w1125, error in (no error)=w1126) -> (element=w1116:dbl[][], error out=w1124:errorcluster)  [unwired: 1 in, 2 out]
            n521 = Enqueue Element(queue=w1130, element="ok", error in (no error)=w1124) -> (error out=w1136:errorcluster)  [unwired: 1 in, 2 out]
            n522 = Dequeue Element(queue=w1137, error in (no error)=w1136) -> (element=w1108:string, error out=w1107:errorcluster)  [unwired: 1 in, 2 out]
            n523 = Equal?(x="stop" ("y"), y=w1108) -> (x = y?=w1110:bool)
            n524 = call "inject_error.vi"("error in"=w1107, "s"=w1110) -> ("error out"=w1106:errorcluster)  [unwired: 9 in]
            n525 = case shown="No Error" w1106 {
              selector: w1106 -> [w1142 w1153]
              tunnel: w1120 -> [w1141 _]
              tunnel: w1119 -> [w1148 _]
              tunnel: w1118 -> [w1147 _]
              tunnel: w1117 -> [w1146 _]
              tunnel: w1116 -> [w1144 _]
              tunnel: w1108 -> [w1143 _]
              tunnel: [w1142 w1153] -> w1105
              frame No Error {
                n526 = Build Path(base path=w1147, name or relative path=w1146) -> (appended path=w1145:path)
                n527 = Match Pattern(string=w1143, regular expression=";") -> (before substring=w1150:string, after substring=w1140:string)  [unwired: 1 in, 2 out]
                n528 = Write to Binary File(file (use dialog)=w1145, data=w1144) -> ()  [unwired: 4 in, 3 out]
                n529 = Build Array(w1146, w1150, w1140, w1141) -> (w1149:string[])
                n530 = call-poly <vilib>:"Write To Spreadsheet File.vi"("append to file? (new file:F)"=TRUE, "1D data"=w1149, "file path (dialog if empty)"=w1148) -> ()  [unwired: 5 in, 1 out]
              }
              frame Error {
              }
            }
          }
          n531 = Dequeue Element(queue=w1077, error in (no error)=w1085) -> (element=w1082:string, error out=w1079:errorcluster)  [unwired: 1 in, 2 out]
          n532 = Equal?(x="stop" ("y"), y=w1082) -> (x = y?=w1080:bool)
          n533 = Or(x=w1080, y=w1079) -> (x .or. y?=w1078:bool)
        }
        n534 = Flush Queue(queue=w1062) -> ()  [unwired: 1 in, 3 out]
      }
      frame "power" {
        w1165 = "stop" ("element")
        w1168 = "start" ("element")
        n535 = local read "meas_voltage"() -> (w1196:i32)
        n536 = Flush Queue(queue=w1206) -> (queue out=w1172:refnum<queue>, error out=w1201:errorcluster)  [unwired: 1 in, 1 out]
        n537 = Flush Queue(queue=w1204) -> (queue out=w1176:refnum<queue>, error out=w1200:errorcluster)  [unwired: 1 in, 1 out]
        n538 = Flush Queue(queue=w1205) -> (queue out=w1174:refnum<queue>, error out=w1199:errorcluster)  [unwired: 1 in, 1 out]
        n539 = Flush Queue(queue=w1203) -> (error out=w1198:errorcluster)  [unwired: 1 in, 2 out]
        n540 = Flush Queue(queue=w1202) -> (queue out=w1175:refnum<queue>, error out=w1197:errorcluster)  [unwired: 1 in, 1 out]
        n541 = local read "header"() -> (w1193:string)
        n542 = Flush Queue(queue=w1162) -> (queue out=w1158:refnum<queue>)  [unwired: 1 in, 2 out]
        n543 = Flush Queue(queue=w1161) -> (queue out=w1160:refnum<queue>)  [unwired: 1 in, 2 out]
        n544 = Merge Errors(w1201, w1200, w1199, w1198, w1197) -> (w1177:errorcluster)
        n545 = local read "Path"() -> (w1207:path)
        n546 = Number To Decimal String(number=w1196) -> (decimal integer string=w1171:string)  [unwired: 1 in]
        n547 = Build Path(base path=w1207, name or relative path=w1193) -> (appended path=w1170:path)
        n548 = Enqueue Element(queue=w1175, element=w1168, error in (no error)=w1177) -> (error out=w1169:errorcluster)  [unwired: 1 in, 2 out]
        n549 = call <vilib>:"Check if File or Folder Exists.vi"("path"=w1170) -> ("file or folder exists?"=w1195:bool, "dup path"=w1194:path)  [unwired: 8 in, 1 out]
        n550 = Enqueue Element(queue=w1158, element=w1168, error in (no error)=w1169) -> (error out=w1167:errorcluster)  [unwired: 1 in, 2 out]
        n551 = case shown="False" w1195 {
          tunnel: [w1212 w1213] -> w1173
          tunnel: w1194 -> [w1211 w1213]
          frame False {
            n552 = Create Folder(path (use dialog)=w1211) -> (created path=w1212:path)  [unwired: 2 in, 2 out]
          }
          frame True {
          }
        }
        n553 = Enqueue Element(queue=w1176, element="snap", error in (no error)=w1167) -> (error out=w1191:errorcluster)  [unwired: 1 in, 2 out]
        n554 = Dequeue Element(queue=w1174, error in (no error)=w1191) -> (element=w1178:dbl[][], error out=w1190:errorcluster)  [unwired: 1 in, 2 out]
        n555 = Enqueue Element(queue=w1175, element=w1165, error in (no error)=w1190) -> (error out=w1166:errorcluster)  [unwired: 1 in, 2 out]
        n556 = Enqueue Element(queue=w1158, element=w1165, error in (no error)=w1166) -> (error out=w1164:errorcluster)  [unwired: 1 in, 2 out]
        n557 = Dequeue Element(queue=w1160, error in (no error)=w1164) -> (element=w1157:dbl[], error out=w1163:errorcluster)  [unwired: 1 in, 2 out]
        n558 = Dequeue Element(queue=w1172, error in (no error)=w1163) -> (element=w1188:string, error out=w1179:errorcluster)  [unwired: 1 in, 2 out]
        n559 = Match Pattern(string=w1188, regular expression=";") -> (before substring=w1186:string, after substring=w1185:string)  [unwired: 1 in, 2 out]
        n560 = flat-sequence {
          tunnel: [w1209] -> w1180
          tunnel: w1179 -> [w1208]
          tunnel: [w1208] -> _
          frame #0 {
            n561 = local read "frames"() -> (w1210:i32)
            n562 = Number To Decimal String(number=w1210) -> (decimal integer string=w1209:string)  [unwired: 1 in]
          }
        }
        n563 = Index Array(array=w1157) -> (element #1=w1156:dbl, element #2=w1155:dbl)  [unwired: 2 in]
        n564 = Format Into String(format string="%.6e_%.6e", w1156, w1155) -> (resulting string=w1159:string)  [unwired: 2 in, 1 out]
        n565 = Format Into String(format string="%s_%s_%s_%s_I%s.bin", w1180, w1171, w1186, w1185, w1159) -> (resulting string=w1184:string)  [unwired: 2 in, 1 out]
        n566 = Build Path(base path=w1173, name or relative path=w1184) -> (appended path=w1183:path)
        n567 = Write to Binary File(file (use dialog)=w1183, data=w1178) -> (refnum out=w1182:refnum<file>, error out=w1181:errorcluster)  [unwired: 4 in, 1 out]
        n568 = Close File(refnum=w1182, error in=w1181) -> ()  [unwired: 2 out]
      }
      frame "power2" {
        n569 = local read "arduino COM"() -> (w1218:refnum<visa-resource-name>)
        n570 = Flush Queue(queue=w1223) -> (queue out=w1229:refnum<queue>, error out=w1237:errorcluster)  [unwired: 1 in, 1 out]
        n571 = Flush Queue(queue=w1222) -> (queue out=w1232:refnum<queue>, error out=w1236:errorcluster)  [unwired: 1 in, 1 out]
        n572 = Flush Queue(queue=w1221) -> (queue out=w1238:refnum<queue>, error out=w1235:errorcluster)  [unwired: 1 in, 1 out]
        n573 = Flush Queue(queue=w1220) -> (error out=w1234:errorcluster)  [unwired: 1 in, 2 out]
        n574 = Flush Queue(queue=w1219) -> (queue out=w1231:refnum<queue>, error out=w1233:errorcluster)  [unwired: 1 in, 1 out]
        n575 = local read "header"() -> (w1224:string)
        n576 = local read "Path"() -> (w1240:path)
        n577 = Merge Errors(w1237, w1236, w1235, w1234, w1233) -> (w1230:errorcluster)
        n578 = Build Path(base path=w1240, name or relative path=w1224) -> (appended path=w1239:path)
        n579 = Build Path(base path=w1239, name or relative path="raw") -> (appended path=w1227:path)
        n580 = call <vilib>:"Check if File or Folder Exists.vi"("path"=w1227) -> ("file or folder exists?"=w1226:bool, "dup path"=w1225:path)  [unwired: 8 in, 1 out]
        n581 = case shown="False" w1226 {
          tunnel: [w1324 w1325] -> w1228
          tunnel: w1225 -> [w1323 w1325]
          frame False {
            n582 = Create Folder(path (use dialog)=w1323) -> (created path=w1324:path)  [unwired: 2 in, 2 out]
          }
          frame True {
          }
        }
        n583 = for {
          N: "powerscan_n" -> [_]
          tunnel: w1238 -> [w1263]
          tunnel: w1232 -> [w1262]
          tunnel: w1231 -> [w1285]
          tunnel: w1230 -> [w1268]
          tunnel: w1229 -> [w1283]
          tunnel: w1228 -> [w1272]
          tunnel: w1218 -> [w1271]
          tunnel: w1216 -> [w1255]
          tunnel: w1215 -> [w1250]
          i -> [w1269]
          n584 = while {
            tunnel: w1268 -> [w1321]
            tunnel: [w1321] -> w1267
            stop <- "pause" continue-if-true
            n585 = case shown="True" "pause" {
              frame False {
              }
              frame True {
                n586 = Wait (ms)(milliseconds to wait=u32 100) -> ()  [unwired: 1 out]
              }
            }
          }
          n587 = local read "arduino_steps"() -> (w1270:i32)
          n588 = call "arduino_mvrel.vi"("error in (no error)"=w1267, "steps"=w1270, "VISA input"=w1271) -> ("error out"=w1261:errorcluster)  [unwired: 6 in, 2 out]
          n589 = case shown="True" "zscan?" {
            tunnel: w1263 -> [_ w1304]
            tunnel: w1262 -> [_ w1303]
            tunnel: w1261 -> [w1290 w1302]
            tunnel: [w1290 w1301] -> w1260
            frame False {
            }
            frame True {
              n590 = local read "IP address"() -> (w1306:string)
              n591 = call "z_opti_rnd.vi"("IP address"=w1306, "range[nm]"="range+-[nm]", "n"="n", "Axis"="Axis", "rand[t] seq [f]"="rand[t] seq [f]", "data"=w1304, "cam"=w1303, "error in (no error)"=w1302) -> ("X"=w1299:dbl[], "Y"=w1300:dbl[], "Best Gaussian Fit"=w1295:dbl[], "error out"=w1301:errorcluster, "center"=→"center":dbl)  [unwired: 3 in]
              n592 = Bundle("X"=w1299, "Y"=w1300) -> (w1297:cluster{"X":dbl[], "Y":dbl[]})  [unwired: 1 in]
              n593 = Bundle("X"=w1299, "Best Gaussian Fit"=w1295) -> (w1298:cluster{"X":dbl[], "Best Gaussian Fit":dbl[]})  [unwired: 1 in]
              n594 = Build Array(w1297, w1298) -> (→"XY Graph 2":cluster{"X":dbl[], "Best Gaussian Fit":dbl[]}[])
            }
          }
          n595 = Enqueue Element(queue=w1285, element="start", error in (no error)=w1260) -> (error out=w1258:errorcluster)  [unwired: 1 in, 2 out]
          n596 = Enqueue Element(queue=w1255, element="start", error in (no error)=w1258) -> (queue out=w1247:refnum<queue>, error out=w1257:errorcluster)  [unwired: 1 in, 1 out]
          n597 = local read "t_exp"() -> (w1243:dbl)
          n598 = Enqueue Element(queue=w1262, element="snap", error in (no error)=w1257) -> (error out=w1288:errorcluster)  [unwired: 1 in, 2 out]
          n599 = Format Into String(format string="%.6e", w1243) -> (resulting string=w1241:string)  [unwired: 2 in, 1 out]
          n600 = Dequeue Element(queue=w1263, error in (no error)=w1288) -> (element=w1264:dbl[][], error out=w1284:errorcluster)  [unwired: 1 in, 2 out]
          n601 = Enqueue Element(queue=w1285, element="stop", error in (no error)=w1284) -> (error out=w1282:errorcluster)  [unwired: 1 in, 2 out]
          n602 = Dequeue Element(queue=w1283, error in (no error)=w1282) -> (element=w1280:string, error out=w1253:errorcluster)  [unwired: 1 in, 2 out]
          n603 = flat-sequence {
            tunnel: [w1318] -> w1266
            tunnel: w1251 -> [w1317]
            tunnel: [w1317] -> w1265
            frame #0 {
              n604 = local read "frames"() -> (w1319:i32)
              n605 = Number To Decimal String(number=w1319) -> (decimal integer string=w1318:string)  [unwired: 1 in]
            }
          }
          n606 = Enqueue Element(queue=w1247, element="stop", error in (no error)=w1253) -> (error out=w1252:errorcluster)  [unwired: 1 in, 2 out]
          n607 = Match Pattern(string=w1280, regular expression=";") -> (before substring=w1278:string, after substring=w1277:string)  [unwired: 1 in, 2 out]
          n608 = Dequeue Element(queue=w1250, error in (no error)=w1252) -> (element=w1246:dbl[], error out=w1251:errorcluster)  [unwired: 1 in, 2 out]
          n609 = Index Array(array=w1246) -> (element #1=w1245:dbl, element #2=w1244:dbl)  [unwired: 2 in]
          n610 = Format Into String(format string="%.6e_%.6e", w1245, w1244) -> (resulting string=w1248:string)  [unwired: 2 in, 1 out]
          n611 = flat-sequence {
            tunnel: w1265 -> [w1316]
            tunnel: [w1316] -> _
            tunnel: w1264 -> [w1315]
            frame #0 {
              n612 = Array Size(array=w1315) -> (size(s)=w1314:i32[])
              n613 = local read "stats"() -> (w1307:dbl)
              n614 = Multiply Array Elements(1:w1314) -> (0:w1312:i32)
              n615 = Add Array Elements(numeric array=w1315) -> (sum=w1313:dbl)
              n616 = Divide(x=w1313, y=w1312) -> (x/y=w1311:dbl)
              n617 = Divide(x=w1307, y=w1311) -> (x/y=w1308:dbl)
              n618 = In Range and Coerce(upper limit=10000.0, x=w1308, lower limit=100.0) -> ()  [unwired: 2 out]
            }
          }
          n619 = Format Into String(format string="%s_%s_%s_%s_I_%s.bin", w1266, w1241, w1278, w1277, w1248) -> (resulting string=w1276:string)  [unwired: 2 in, 1 out]
          n620 = Build Path(base path=w1272, name or relative path=w1276) -> (appended path=w1275:path)
          n621 = Write to Binary File(file (use dialog)=w1275, data=w1264) -> (refnum out=w1274:refnum<file>, error out=w1273:errorcluster)  [unwired: 4 in, 1 out]
          n622 = Close File(refnum=w1274, error in=w1273) -> ()  [unwired: 2 out]
          "prog" <- w1269
        }
      }
      frame "delay" {
        n623 = local read "Path"() -> (w1345:path)
        n624 = Dequeue Element(queue=w1332) -> ()  [unwired: 2 in, 4 out]
        n625 = Build Path(base path=w1345, name or relative path="delayscan_header") -> (appended path=w1334:path)
        n626 = call <vilib>:"Check if File or Folder Exists.vi"("path"=w1334) -> ("file or folder exists?"=w1336:bool, "dup path"=w1335:path)  [unwired: 8 in, 1 out]
        n627 = case shown="False" w1336 {
          tunnel: [w1460 w1461] -> w1333
          tunnel: w1335 -> [w1459 w1461]
          frame False {
            n628 = Create Folder(path (use dialog)=w1459) -> (created path=w1460:path)  [unwired: 2 in, 2 out]
          }
          frame True {
          }
        }
        n629 = call "create scan vectr.vi"("Table Control"="waypoints") -> ("Array"=w1337:dbl[])
        n630 = Flush Queue(queue=w1330) -> (queue out=w1331:refnum<queue>)  [unwired: 1 in, 2 out]
        n631 = Array Size(array=w1337) -> (size(s)=w1340:i32)
        n632 = Build Path(base path=w1333, name or relative path="times.txt") -> (appended path=w1342:path)
        n633 = Flush Queue(queue=w1327) -> (queue out=w1326:refnum<queue>)  [unwired: 1 in, 2 out]
        n634 = Flush Queue(queue=w1329) -> (queue out=w1328:refnum<queue>)  [unwired: 1 in, 2 out]
        n635 = Initialize Array(0.0 ("element"), w1340) -> (w1338:dbl[])
        n636 = call-poly <vilib>:"Write To Spreadsheet File.vi"("transpose? (no:F)"=TRUE, "1D data"=w1337, "file path (dialog if empty)"=w1342) -> ()  [unwired: 5 in, 1 out]
        n637 = while {
          tunnel: w1337 -> [w1358]
          tunnel: w1326 -> [w1362]
          tunnel: w1346 -> [w1361]
          tunnel: w1331 -> [w1360]
          tunnel: w1328 -> [w1359]
          tunnel: w1333 -> [w1357]
          shift-right: [w1355] -> _
          shift-left: w1338 -> [w1356]
          tunnel: w1333 -> [w1354]
          i -> [w1351]
          stop <- w1348 stop-if-true
          n638 = for {
            tunnel: w1358 -> [w1373] mode=indexing
            tunnel: w1362 -> [w1447]
            tunnel: w1361 -> [w1445]
            tunnel: w1360 -> [w1443]
            tunnel: w1359 -> [w1441]
            tunnel: w1358 -> [w1411]
            tunnel: w1357 -> [w1439]
            tunnel: w1351 -> [w1371]
            shift-right: [w1409] -> w1355
            shift-left: w1356 -> [w1412]
            tunnel: w1354 -> [w1407]
            tunnel: ["delayscan_stop"] -> w1350
            i -> [w1377]
            stop <- "delayscan_stop" stop-if-true
            w1402 = T3 7 items=["Grayscale (U8)", "Grayscale (I16)", "Grayscale (SGL)", "Complex (CSG)", "RGB (U32)", "HSL (U32)", "RGB (U64)", "Grayscale (U16)"] ("Image Type")
            n639 = local read "t0 @"() -> (w1452:dbl)
            n640 = Get Date/Time In Seconds() -> (seconds since 1Jan1904=w1367:timestamp)
            n641 = Divide(x=w1371, y=10000) -> (x/y=w1437:dbl)
            n642 = Negate(x=w1373) -> (-x=w1374:dbl)
            n643 = Format Date/Time String(time format string (%c)="DelayScan_%Y%m%d_%H%M%S_", seconds (now)=w1367) -> (date/time string=w1363:string)  [unwired: 1 in]
            n644 = Divide(x=w1377, y=10000) -> (x/y=w1376:dbl)
            n645 = Number To Fractional String(number=w1437) -> (F-format string=w1436:string)  [unwired: 3 in]
            n646 = call "time2mm.vi"("fs[1]/ps[0]"=TRUE, "Offset (mm)"=w1452, "time"=w1374) -> ("position (mm)"=w1370:dbl)
            n647 = Number To Fractional String(number=w1376) -> (F-format string=w1432:string)  [unwired: 3 in]
            n648 = Number To Fractional String(number=w1370) -> (F-format string=w1450:string)  [unwired: 3 in]
            n649 = String Subset(string=w1436, offset (0)=2, length (rest)=4 ("length (rest)")) -> (substring=w1434:string)
            n650 = String Subset(string=w1432, offset (0)=2, length (rest)=4 ("length (rest)")) -> (substring=w1365:string)
            n651 = Concatenate Strings("abs:" ("string"), w1450, ":confirm" ("string")) -> (w1448:string)
            n652 = Build Path(base path=w1439, name or relative path=w1434) -> (appended path=w1380:path)
            n653 = call <vilib>:"Check if File or Folder Exists.vi"("path"=w1380) -> ("file or folder exists?"=w1381:bool, "dup path"=w1382:path)  [unwired: 8 in, 1 out]
            n654 = Concatenate Strings(w1363, w1365) -> (w1366:string)
            n655 = case shown="False" w1381 {
              tunnel: [w1455 w1456] -> w1379
              tunnel: w1382 -> [w1454 w1456]
              frame False {
                n656 = Create Folder(path (use dialog)=w1454) -> (created path=w1455:path)  [unwired: 2 in, 2 out]
              }
              frame True {
              }
            }
            n657 = Enqueue Element(queue=w1447, element=w1448) -> (error out=w1446:errorcluster)  [unwired: 2 in, 2 out]
            n658 = Concatenate Strings(w1366, ".bin" ("string")) -> (w1387:string)
            n659 = Concatenate Strings(w1366, ".png" ("string")) -> (w1385:string)
            n660 = Wait on Notification(notifier=w1445, error in (no error)=w1446) -> (error out=w1444:errorcluster)  [unwired: 2 in, 3 out]
            n661 = Build Path(base path=w1379, name or relative path=w1387) -> (appended path=w1408:path)
            n662 = Build Path(base path=w1407, name or relative path="positions.txt") -> (appended path=w1405:path)
            n663 = property on="live" class="IntGraph (strict)"() -> ("CrsrLis"=w1431:T9)  [unwired: 2 in, 2 out]
            n664 = Build Path(base path=w1379, name or relative path=w1385) -> (appended path=w1384:path)
            n665 = Enqueue Element(queue=w1441, element="snap", error in (no error)=w1444) -> (error out=w1442:errorcluster)  [unwired: 1 in, 2 out]
            n666 = Index Array(array=w1431) -> (element #1=w1430:T10, element #2=w1429:T10)  [unwired: 2 in]
            n667 = Unbundle By Name(w1430) -> ("Position.X"=w1428:dbl, "Position.Y"=w1426:dbl)
            n668 = Unbundle By Name(w1429) -> ("Position.X"=w1427:dbl, "Position.Y"=w1425:dbl)
            n669 = Dequeue Element(queue=w1443, error in (no error)=w1442) -> (element=w1383:dbl[][])  [unwired: 1 in, 3 out]
            n670 = Build Array(w1428, w1427) -> (w1424:dbl[])
            n671 = Build Array(w1426, w1425) -> (w1423:dbl[])
            n672 = Array Max & Min(array=w1424) -> (max value=w1422:dbl, min value=w1420:dbl)  [unwired: 2 out]
            n673 = Array Max & Min(array=w1423) -> (max value=w1421:dbl, min value=w1418:dbl)  [unwired: 2 out]
            n674 = Write to Binary File(file (use dialog)=w1408, data=w1383) -> ()  [unwired: 4 in, 3 out]
            n675 = Subtract(x=w1420, y=w1422) -> (x-y=w1419:dbl)
            n676 = Subtract(x=w1418, y=w1421) -> (x-y=w1417:dbl)
            n677 = Array Subset(array=w1383, index (row)=w1420, length (row)=w1419, index (col)=w1418, length (col)=w1417) -> (w1416:dbl[][])
            n678 = Array Size(array=w1383) -> (size(s)=w1414:i32[])
            n679 = Add Array Elements(numeric array=w1416) -> (sum=w1415:dbl)
            n680 = Multiply Array Elements(1:w1414) -> (0:w1413:i32)
            n681 = Divide(x=w1415, y=w1413) -> ()  [unwired: 1 out]
            n682 = for {
              tunnel: w1383 -> [w1458] mode=indexing
              tunnel: [w1457] -> w1397 mode=indexing
              n683 = Reverse 1D Array(array=w1458) -> (reversed array=w1457:dbl[])
            }
            n684 = Replace Array Subset(array=w1412, new element=w1370, index=w1377) -> (w1409:dbl[])
            n685 = Bundle("Array"=w1411, w1409) -> (→"XY Graph":cluster{"Array":dbl[], dbl[]})  [unwired: 1 in]
            n686 = call-poly <vilib>:"Write To Spreadsheet File.vi"("transpose? (no:F)"=TRUE, "format (%.3f)"="%.6f", "1D data"=w1409, "file path (dialog if empty)"=w1405) -> ()  [unwired: 4 in, 1 out]
            n687 = Transpose 2D Array(2D array=w1397) -> (transposed array=w1391:dbl[][])
            n688 = Array Max & Min(array=w1391) -> (min value=w1390:dbl)  [unwired: 3 out]
            n689 = Subtract(x=w1391, y=w1390) -> (x-y=w1389:dbl[][])
            n690 = call "IMAQ Create"("Image Name"="untitled", "Image Type"=w1402) -> ("New Image"=w1403:T4)  [unwired: 3 in, 1 out]
            n691 = Array Max & Min(array=w1389) -> (max value=w1396:dbl)  [unwired: 3 out]
            n692 = Divide(x=w1389, y=w1396) -> (x/y=w1395:dbl[][])
            n693 = Multiply(x=w1395, y=255) -> (x*y=w1393:dbl[][])
            n694 = To Unsigned Word Integer(number=w1393) -> (unsigned 16bit integer=w1392:u16[][])
            n695 = call "IMAQ ArrayToImage"("Image Pixels (U16)"=w1392, "Image"=w1403) -> ("Image Out"=w1401:T4)  [unwired: 8 in, 1 out]
            n696 = call-poly "IMAQ Write File 2"("Image Quality"=u32 1000, "File Path"=w1384, "Image"=w1401) -> ("Image Out (duplicate)"=w1399:T4)  [unwired: 7 in, 1 out]
            n697 = call "IMAQ Dispose"("Image"=w1399) -> ()  [unwired: 5 in, 1 out]
          }
          n698 = Increment(x=w1351) -> (x+1=w1352:i32)
          n699 = Greater Or Equal?(x=w1352, y="iterations") -> (x >= y?=w1349:bool)
          n700 = Or(x=w1350, y=w1349) -> (x .or. y?=w1348:bool)
        }
      }
      frame "idle", Default {
      }
    }
  }
  n701 = Set Occurrence(w12) -> ()
